vi "MAIN.vi"() -> ()   [LabVIEW 2021]
doc: "This is the main VI of the program. \n\nThis program required devices: the Power Meter (PM), the Stepper Motor (SM) and the Scannners."
uses:
  State.ctl
  State_2.ctl
  Data.ctl
  camera_data_cluster.ctl
  <vilib>/Utility/error.llb/DialogType.ctl
  <vilib>/DAQmx/write.llb/DAQmx Write (Analog 2D DBL NChan NSamp).vi
  <vilib>/DAQmx/read.llb/DAQmx Read (Digital Bool 1Line 1Point).vi
  <vilib>/DAQmx/create/channels.llb/DAQmx Create Channel (AO-Voltage-Basic).vi
  <vilib>/DAQmx/create/channels.llb/DAQmx Create Channel (DI-Digital Input).vi
  <vilib>/DAQmx/configure/timing.llb/DAQmx Timing (Sample Clock).vi
  <vilib>/DAQmx/miscellaneous.llb/DAQmx Fill In Error Info.vi
panel:
  out "Init filter position":sgl
  in  "Filter":bool
  out "FIX SM MotorRunState":i32(ring) items=["RunUnspecified", "RunStop", "RunForward", "RunReverse"]
  out "FIX SM CurrPosition":sgl
  out "FIX SM FaultStatus":bool
  out "IR SM MotorRunState":i32(ring) items=["RunUnspecified", "RunStop", "RunForward", "RunReverse"]
  out "IR SM CurrPosition":sgl
  out "IR SM FaultStatus":bool
  out "VIS SM MotorRunState":i32(ring) items=["RunUnspecified", "RunStop", "RunForward", "RunReverse"]
  out "VIS SM CurrPosition":sgl
  out "VIS SM FaultStatus":bool
  out "VIS GF MotorRunState":i32(ring) items=["RunUnspecified", "RunStop", "RunForward", "RunReverse"]
  out "VIS GF CurrPosition":sgl
  out "VIS GF FaultStatus":bool
  out "IR GF MotorRunState":i32(ring) items=["RunUnspecified", "RunStop", "RunForward", "RunReverse"]
  out "IR GF CurrPosition":sgl
  out "IR GF FaultStatus":bool
  out "Enum":T1=enum."Set power_1"
  in  "Threshold finding step [dB]":dbl=0.35 caption="Init power level [W]"
  in  "Investigated brightness range [dB]":sgl=10.0 caption="Init power level [W]"
  in  "Number of points M-2":i32=10 caption="Init power level [W]"
  in  "Number of trials k":i32=10 caption="Init power level [W]"
  out "Camera Image":picture
  out "Intensity graph output image":u8[][](graph) caption="Intensity Graph"
  out "error out 2":errorcluster
  out "loop down cond.":bool=TRUE
  out "loop up cond.":bool=TRUE
  out "Previous Position":i32=16
  in  "Save image?":bool
  out "#elements in queue":i32=2626
  out "Number of saved images":i32=2626
  in  "N_pts":u8=255
  in  "img_cols":u16=600
  in  "GB":u8=15
  in  "img_rows":u16=600
  in  "AT":u8=21
  in  "Auto gain":bool
  in  "Gain":i32(slide) scale=0.0..100.0
  in  "Frame rate":dbl(slide)=10.000850072256142 scale=9.830199684122917..40.10842644615945
  in  "Pixel clock":i32(slide)=24 scale=5.0..43.0
  in  "Exposure time":dbl(slide)=99.92475 scale=0.03841666666666667..99.96016666666667
  out "C brightness":bool[](array[boolean])
  out "Found?":bool[](array[boolean])=[TRUE, TRUE, TRUE, TRUE, TRUE, TRUE, TRUE, TRUE, TRUE, TRUE, TRUE, TRUE, TRUE, TRUE, TRUE, TRUE, TRUE]
  in  "Set Min Power [W]":dbl=8e-07 caption="Wavelength (0.0)" format="%#_6p"
  in  "Stop program":bool
  in  "Init power level [W]":dbl=0.0004 format="%#_6p"
  out "Measur. start time":timestamp=timestamp(3662016175.3575897 s since 1904-01-01)
  in  "Menu":enum32{"Test mode", "Measurement"}(tab)=enum."Measurement"
  in  "VIS SM GTP":bool
  in  "IR SM GTP":bool
  in  "FIX SM GTP":bool
  in  "VIS SM GTP":bool
  in  "IR SM GTP":bool
  in  "VIS GF GoToPos":sgl
  in  "IR GF GoToPos":sgl
  in  "FIX SM GoToPos":sgl
  in  "VIS SM GoToPos":sgl
  in  "IR SM GoToPos":sgl
  in  "Stimulus":bool
  in  "Illuminator OFF":bool
  in  "VIS br SM step [deg]":sgl
  in  "IR br SM step [deg]":sgl
  in  "FIX ref SM step [mm]":sgl
  in  "VIS ref SM step [mm]":sgl
  in  "IR ref SM step [mm]":sgl
  in  "VIS shutter":bool
  in  "IR shutter":bool
  in  "VIS brightness":bool
  in  "IR brightness":bool
  in  "FIX refraction SM":bool
  in  "VIS refraction SM":bool
  in  "IR refraction SM":bool
  in  "OK Button 2":bool
  in  "Set power [W]":dbl=6e-07 format="%#_6p"
  in  "FIX OFF":bool
  out "Test optotype":cluster{"sine wave":dbl[], "sine wave":dbl[]}(graph)={"sine wave"=[0.0, 0.002453383716370901, 0.0049008570164780305, 0.007336523722768088, 0.009754516100806413, 0.012149008995163194, 0.014514233862723118, 0.016844492669611, 0.019134171618254488, 0.021377754671514104, 0.02356983684129988, 0.025705137209661083, 0.02777851165098011, 0.029784965224621665, 0.03171966420818227, 0.03357794774235092, 0.035355339059327376, 0.03704755626774796, 0.038650522668136844, 0.04016037657403225, 0.04157348061512726, 0.04288643050001361, 0.04409606321741775, 0.045199464656172174, 0.046193976625564334, 0.047077203259151046, 0.047847016786610436, 0.04850156265972721, 0.04903926402016152, 0.04945882549823906, 0.04975923633360984, 0.04993977281025863, 0.049999999999999996, 0.04993977281025863, 0.04975923633360984, 0.04945882549823906, 0.04903926402016152, 0.04850156265972721, 0.047847016786610436, 0.047077203259151046, 0.04619397662556433, 0.045199464656172174, 0.04409606321741774, 0.04288643050001361, 0.04157348061512725, 0.04016037657403225, 0.03865052266813684, 0.03704755626774796, 0.03535533905932737, 0.03357794774235092, 0.03171966420818227, 0.029784965224621665, 0.02777851165098011, 0.025705137209661083, 0.02356983684129988, 0.0213777546715141, 0.019134171618254488, 0.016844492669610998, 0.014514233862723118, 0.012149008995163189, 0.009754516100806413, 0.007336523722768081, 0.00490085701647803, 0.002453383716370893, 0.0, -0.0024533837163709096, -0.00490085701647803, -0.007336523722768097, -0.009754516100806413, -0.012149008995163205, -0.014514233862723117, -0.016844492669611015, -0.019134171618254488, -0.021377754671514117, -0.02356983684129988, -0.0257051372096611, -0.02777851165098011, -0.029784965224621682, -0.03171966420818227, -0.033577947742350935, -0.03535533905932737, -0.03704755626774797, -0.03865052266813684, -0.040160376574032264, -0.04157348061512725, -0.042886430500013624, -0.04409606321741774, -0.04519946465617219, -0.04619397662556433, -0.04707720325915106, -0.047847016786610436, -0.04850156265972722, -0.04903926402016152, -0.04945882549823907, -0.04975923633360984, -0.049939772810258645, -0.049999999999999996, -0.049939772810258645, -0.04975923633360984, -0.04945882549823907, -0.04903926402016152, -0.04850156265972722, -0.047847016786610436, -0.04707720325915106, -0.04619397662556433, -0.04519946465617219, -0.04409606321741774, -0.042886430500013624, -0.04157348061512725, -0.040160376574032264, -0.03865052266813684, -0.03704755626774797, -0.03535533905932737, -0.033577947742350935, -0.03171966420818227, -0.02978496522462168, -0.02777851165098011, -0.025705137209661093, -0.02356983684129988, -0.021377754671514107, -0.019134171618254488, -0.016844492669611, -0.014514233862723118, -0.012149008995163189, -0.009754516100806413, -0.007336523722768078, -0.00490085701647803, -0.002453383716370887], "sine wave"=[0.05, 0.049939772810258624, 0.049759236333609846, 0.04945882549823905, 0.049039264020161524, 0.0485015626597272, 0.04784701678661044, 0.04707720325915104, 0.046193976625564334, 0.04519946465617217, 0.04409606321741775, 0.0428864305000136, 0.04157348061512726, 0.04016037657403224, 0.038650522668136844, 0.03704755626774795, 0.035355339059327376, 0.033577947742350914, 0.03171966420818227, 0.02978496522462166, 0.02777851165098011, 0.025705137209661083, 0.02356983684129988, 0.0213777546715141, 0.019134171618254488, 0.016844492669610998, 0.014514233862723117, 0.01214900899516319, 0.00975451610080641, 0.007336523722768084, 0.004900857016478025, 0.0024533837163708975, -6.071532165918825e-18, -0.0024533837163709035, -0.0049008570164780375, -0.00733652372276809, -0.009754516100806422, -0.012149008995163198, -0.014514233862723127, -0.016844492669611005, -0.019134171618254498, -0.021377754671514107, -0.023569836841299895, -0.025705137209661087, -0.027778511650980123, -0.029784965224621665, -0.031719664208182285, -0.033577947742350914, -0.03535533905932739, -0.037047556267747944, -0.03865052266813686, -0.040160376574032236, -0.04157348061512727, -0.042886430500013596, -0.04409606321741776, -0.04519946465617216, -0.04619397662556435, -0.04707720325915103, -0.04784701678661045, -0.048501562659727195, -0.04903926402016153, -0.049458825498239045, -0.04975923633360985, -0.04993977281025862, -0.05, -0.04993977281025862, -0.049759236333609846, -0.049458825498239045, -0.049039264020161524, -0.048501562659727195, -0.04784701678661044, -0.04707720325915103, -0.046193976625564334, -0.04519946465617216, -0.04409606321741775, -0.042886430500013596, -0.04157348061512726, -0.040160376574032236, -0.038650522668136844, -0.037047556267747944, -0.03535533905932737, -0.033577947742350914, -0.031719664208182265, -0.02978496522462166, -0.0277785116509801, -0.025705137209661083, -0.023569836841299867, -0.021377754671514104, -0.01913417161825447, -0.016844492669611, -0.0145142338627231, -0.012149008995163194, -0.009754516100806392, -0.007336523722768088, -0.004900857016478009, -0.002453383716370901, 2.168404344971009e-17, 0.0024533837163709, 0.004900857016478052, 0.007336523722768087, 0.009754516100806436, 0.012149008995163194, 0.01451423386272314, 0.016844492669611, 0.019134171618254512, 0.021377754671514104, 0.023569836841299905, 0.025705137209661083, 0.027778511650980133, 0.02978496522462166, 0.0317196642081823, 0.033577947742350914, 0.035355339059327404, 0.037047556267747944, 0.03865052266813687, 0.040160376574032236, 0.041573480615127285, 0.042886430500013596, 0.044096063217417776, 0.04519946465617216, 0.04619397662556436, 0.04707720325915103, 0.04784701678661046, 0.048501562659727195, 0.04903926402016154, 0.049458825498239045, 0.04975923633360986, 0.04993977281025862]}
  in  "Hide optotype":bool
  in  "X position":dbl
  in  "Select test optotype":u16(ring)=3 caption="Select optotype" items=["Circle", "Cross", "Square", "Flicker circle", "Beam", "Flicker beam"]
  in  "Y position":dbl
  in  "Size [V]":dbl=0.05 format="%#_13g"
  out "Threshold found?":bool
  out "Progress - found locations":u8(slide) max=5 step=1 scale=0.0..120.0
  in  "NO button":bool
  in  "YES button":bool
  out "Rate":dbl=12800.0
  in  "Min/Max Voltage":dbl=0.05 format="%#_13g"
  out "XY Graph":cluster{"sine wave":dbl[], "sine wave":dbl[]}(graph)={"sine wave"=[0.0, 0.002453383716370901, 0.0049008570164780305, 0.007336523722768088, 0.009754516100806413, 0.012149008995163194, 0.014514233862723118, 0.016844492669611, 0.019134171618254488, 0.021377754671514104, 0.02356983684129988, 0.025705137209661083, 0.02777851165098011, 0.029784965224621665, 0.03171966420818227, 0.03357794774235092, 0.035355339059327376, 0.03704755626774796, 0.038650522668136844, 0.04016037657403225, 0.04157348061512726, 0.04288643050001361, 0.04409606321741775, 0.045199464656172174, 0.046193976625564334, 0.047077203259151046, 0.047847016786610436, 0.04850156265972721, 0.04903926402016152, 0.04945882549823906, 0.04975923633360984, 0.04993977281025863, 0.049999999999999996, 0.04993977281025863, 0.04975923633360984, 0.04945882549823906, 0.04903926402016152, 0.04850156265972721, 0.047847016786610436, 0.047077203259151046, 0.04619397662556433, 0.045199464656172174, 0.04409606321741774, 0.04288643050001361, 0.04157348061512725, 0.04016037657403225, 0.03865052266813684, 0.03704755626774796, 0.03535533905932737, 0.03357794774235092, 0.03171966420818227, 0.029784965224621665, 0.02777851165098011, 0.025705137209661083, 0.02356983684129988, 0.0213777546715141, 0.019134171618254488, 0.016844492669610998, 0.014514233862723118, 0.012149008995163189, 0.009754516100806413, 0.007336523722768081, 0.00490085701647803, 0.002453383716370893, 0.0, -0.0024533837163709096, -0.00490085701647803, -0.007336523722768097, -0.009754516100806413, -0.012149008995163205, -0.014514233862723117, -0.016844492669611015, -0.019134171618254488, -0.021377754671514117, -0.02356983684129988, -0.0257051372096611, -0.02777851165098011, -0.029784965224621682, -0.03171966420818227, -0.033577947742350935, -0.03535533905932737, -0.03704755626774797, -0.03865052266813684, -0.040160376574032264, -0.04157348061512725, -0.042886430500013624, -0.04409606321741774, -0.04519946465617219, -0.04619397662556433, -0.04707720325915106, -0.047847016786610436, -0.04850156265972722, -0.04903926402016152, -0.04945882549823907, -0.04975923633360984, -0.049939772810258645, -0.049999999999999996, -0.049939772810258645, -0.04975923633360984, -0.04945882549823907, -0.04903926402016152, -0.04850156265972722, -0.047847016786610436, -0.04707720325915106, -0.04619397662556433, -0.04519946465617219, -0.04409606321741774, -0.042886430500013624, -0.04157348061512725, -0.040160376574032264, -0.03865052266813684, -0.03704755626774797, -0.03535533905932737, -0.033577947742350935, -0.03171966420818227, -0.02978496522462168, -0.02777851165098011, -0.025705137209661093, -0.02356983684129988, -0.021377754671514107, -0.019134171618254488, -0.016844492669611, -0.014514233862723118, -0.012149008995163189, -0.009754516100806413, -0.007336523722768078, -0.00490085701647803, -0.002453383716370887], "sine wave"=[0.05, 0.049939772810258624, 0.049759236333609846, 0.04945882549823905, 0.049039264020161524, 0.0485015626597272, 0.04784701678661044, 0.04707720325915104, 0.046193976625564334, 0.04519946465617217, 0.04409606321741775, 0.0428864305000136, 0.04157348061512726, 0.04016037657403224, 0.038650522668136844, 0.03704755626774795, 0.035355339059327376, 0.033577947742350914, 0.03171966420818227, 0.02978496522462166, 0.02777851165098011, 0.025705137209661083, 0.02356983684129988, 0.0213777546715141, 0.019134171618254488, 0.016844492669610998, 0.014514233862723117, 0.01214900899516319, 0.00975451610080641, 0.007336523722768084, 0.004900857016478025, 0.0024533837163708975, -6.071532165918825e-18, -0.0024533837163709035, -0.0049008570164780375, -0.00733652372276809, -0.009754516100806422, -0.012149008995163198, -0.014514233862723127, -0.016844492669611005, -0.019134171618254498, -0.021377754671514107, -0.023569836841299895, -0.025705137209661087, -0.027778511650980123, -0.029784965224621665, -0.031719664208182285, -0.033577947742350914, -0.03535533905932739, -0.037047556267747944, -0.03865052266813686, -0.040160376574032236, -0.04157348061512727, -0.042886430500013596, -0.04409606321741776, -0.04519946465617216, -0.04619397662556435, -0.04707720325915103, -0.04784701678661045, -0.048501562659727195, -0.04903926402016153, -0.049458825498239045, -0.04975923633360985, -0.04993977281025862, -0.05, -0.04993977281025862, -0.049759236333609846, -0.049458825498239045, -0.049039264020161524, -0.048501562659727195, -0.04784701678661044, -0.04707720325915103, -0.046193976625564334, -0.04519946465617216, -0.04409606321741775, -0.042886430500013596, -0.04157348061512726, -0.040160376574032236, -0.038650522668136844, -0.037047556267747944, -0.03535533905932737, -0.033577947742350914, -0.031719664208182265, -0.02978496522462166, -0.0277785116509801, -0.025705137209661083, -0.023569836841299867, -0.021377754671514104, -0.01913417161825447, -0.016844492669611, -0.0145142338627231, -0.012149008995163194, -0.009754516100806392, -0.007336523722768088, -0.004900857016478009, -0.002453383716370901, 2.168404344971009e-17, 0.0024533837163709, 0.004900857016478052, 0.007336523722768087, 0.009754516100806436, 0.012149008995163194, 0.01451423386272314, 0.016844492669611, 0.019134171618254512, 0.021377754671514104, 0.023569836841299905, 0.025705137209661083, 0.027778511650980133, 0.02978496522462166, 0.0317196642081823, 0.033577947742350914, 0.035355339059327404, 0.037047556267747944, 0.03865052266813687, 0.040160376574032236, 0.041573480615127285, 0.042886430500013596, 0.044096063217417776, 0.04519946465617216, 0.04619397662556436, 0.04707720325915103, 0.04784701678661046, 0.048501562659727195, 0.04903926402016154, 0.049458825498239045, 0.04975923633360986, 0.04993977281025862]}
  in  "Select optotype":u16(ring)=3 items=["Circle", "Cross", "Square", "Flicker circle", "Beam", "Flicker beam"]
  in  "shiftX":dbl
  in  "shiftY":dbl
  in  "Start measurement":bool
  in  "Pause":bool
  out "Answers":i32[][](array[numeric])
  out "Previous brightess":i32
  out "Filter positions [deg]":sgl[](array[numeric])
  out "Progress - found locations 2":u8 max=5 step=1
  in  "Set Max Power [W]":dbl=0.0004 caption="Wavelength (0.0)" format="%#_6p"
  out "Patient button":bool
  out "Any USB device connected?":bool=TRUE
  in  "Set Wavelength [nm]":dbl=1040.0 caption="Wavelength (0.0)"
  out "Current position [steps]":i32
  in  "File Path":path=path "D:/meas_data"
  out "Power Value":dbl=4.76676519e-07 caption="Optical Power [W]" format="%#_4p"
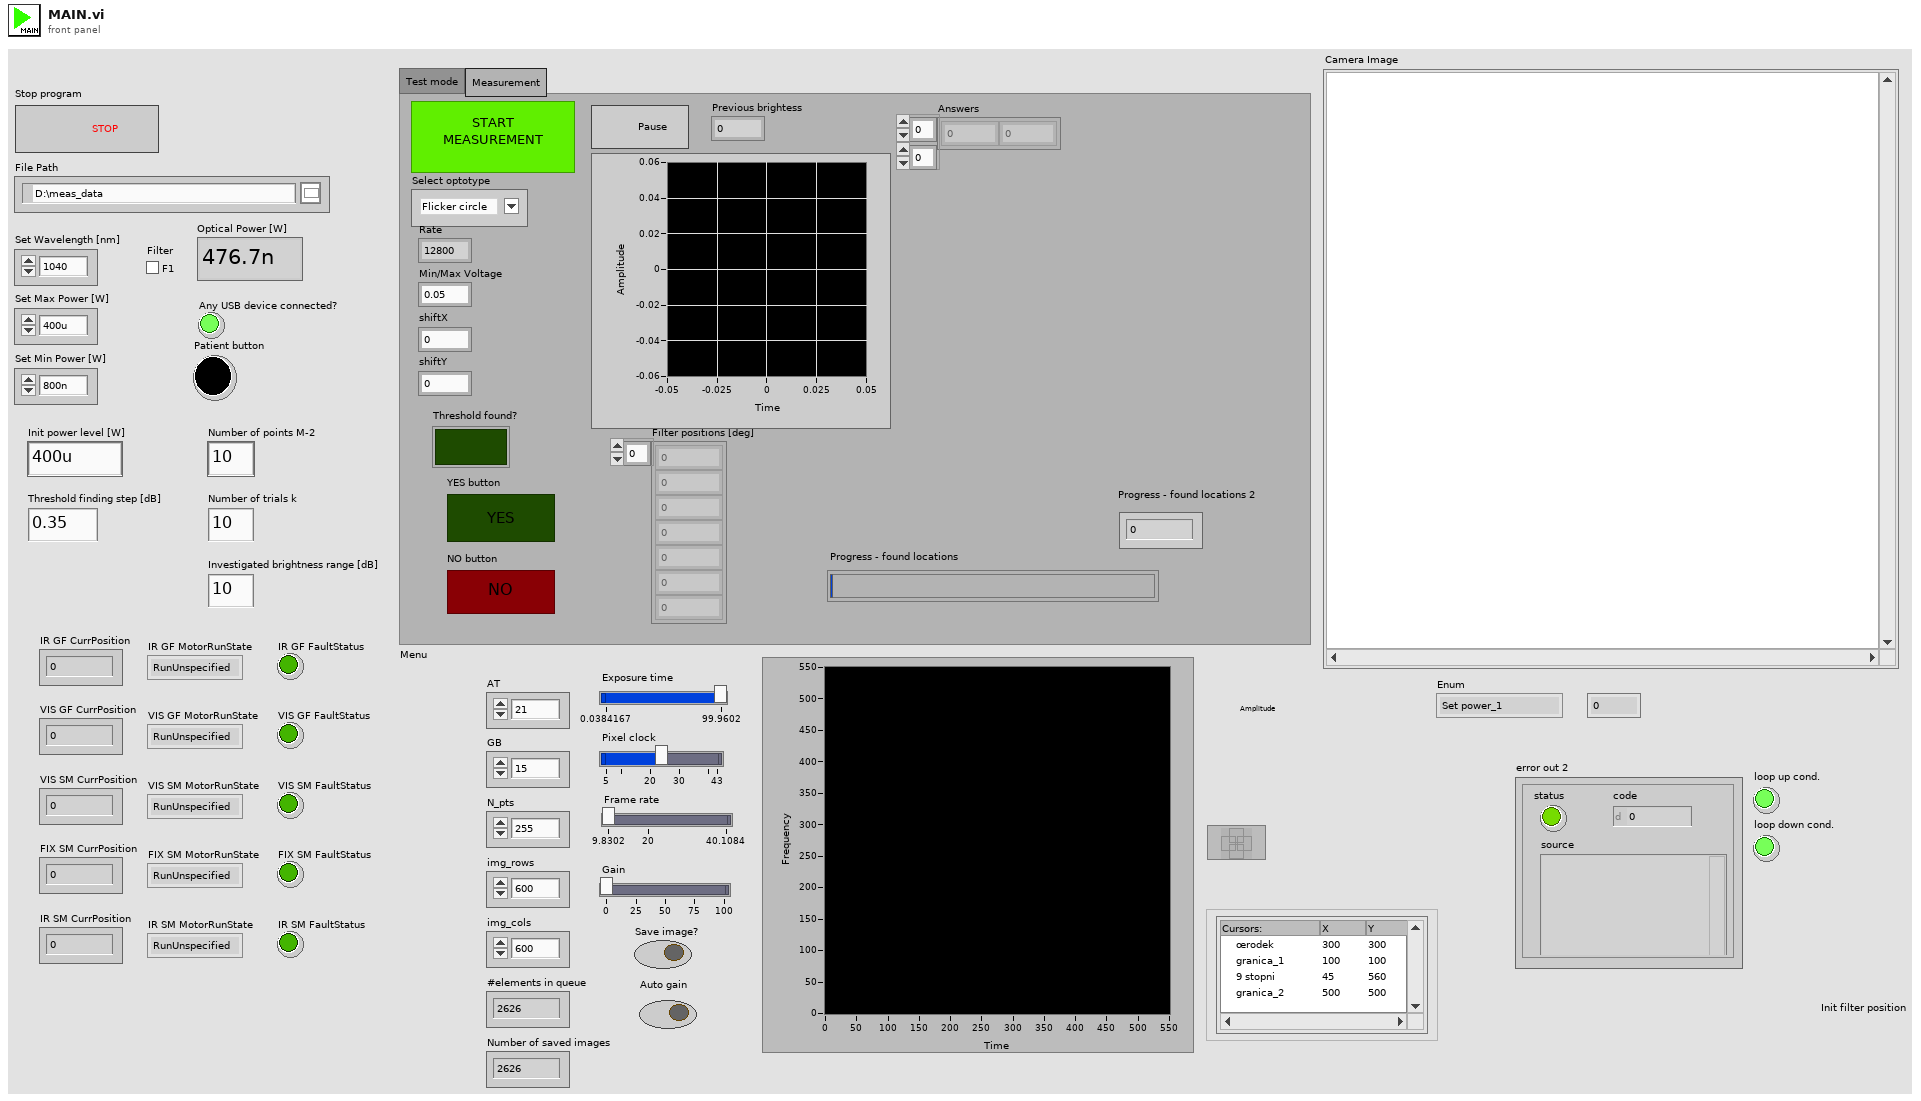
[diagram p1: front panel]
types:
  T1 = typedef "State.ctl" = enum16{"Initialize", "Idle_2", "Random brightness", "Hide optotype_2", "Hide optotype_1", "Set power_1", "Set_power_2", "Show optotype", "Wait for event", "Yes_1", "Yes_2", "No_2", "No_1", "Idle_1", "Exit"}
  T2 = typedef "Data.ctl" = cluster{cluster{"Power [W]":dbl, "Position":string, "Answer":string, "Seconds form start [s]":dbl, "Time stamp":timestamp}}[]
  T3 = typedef "State_2.ctl" = enum16{"Wait for event", "Set power", "Update optotype"}
  T4 = typedef "camera_data_cluster.ctl" = cluster{"Time stamp":timestamp, "Image":u8[][], "Z Scale.Range:Maximum":dbl, "Z Scale.Range:Minimum":dbl, "Color Table":u32[]}
  T5 = cluster{"s32Width":i32, "s32PosX":i32, "s32PosY":i32, "s32PosY":i32}
  T6 = cluster{"Power Value":dbl, string, string, dbl, "seconds since 1Jan1904":timestamp}
  T7 = cluster{cluster{"Power Value":dbl, string, string, dbl, "seconds since 1Jan1904":timestamp}}[]
  T8 = cluster{"Pixel clock":refnum<vi>, "Frame rate":refnum<vi>, "Exposure time":refnum<vi>, "Gain":refnum<vi>, "Auto gain":bool}
  T9 = cluster{"img_rows":u16, "img_cols":u16, "AT":u8, "GB":u8, "N_pts":u8}
  T10 = typedef "DialogType.ctl" = u16
  T11 = cluster{"Set Wavelength [nm]":dbl, "Min/Max Voltage":dbl, "shiftX":dbl, "shiftY":dbl, "Filter positions [deg]":sgl[], "Answers":i32[][]}
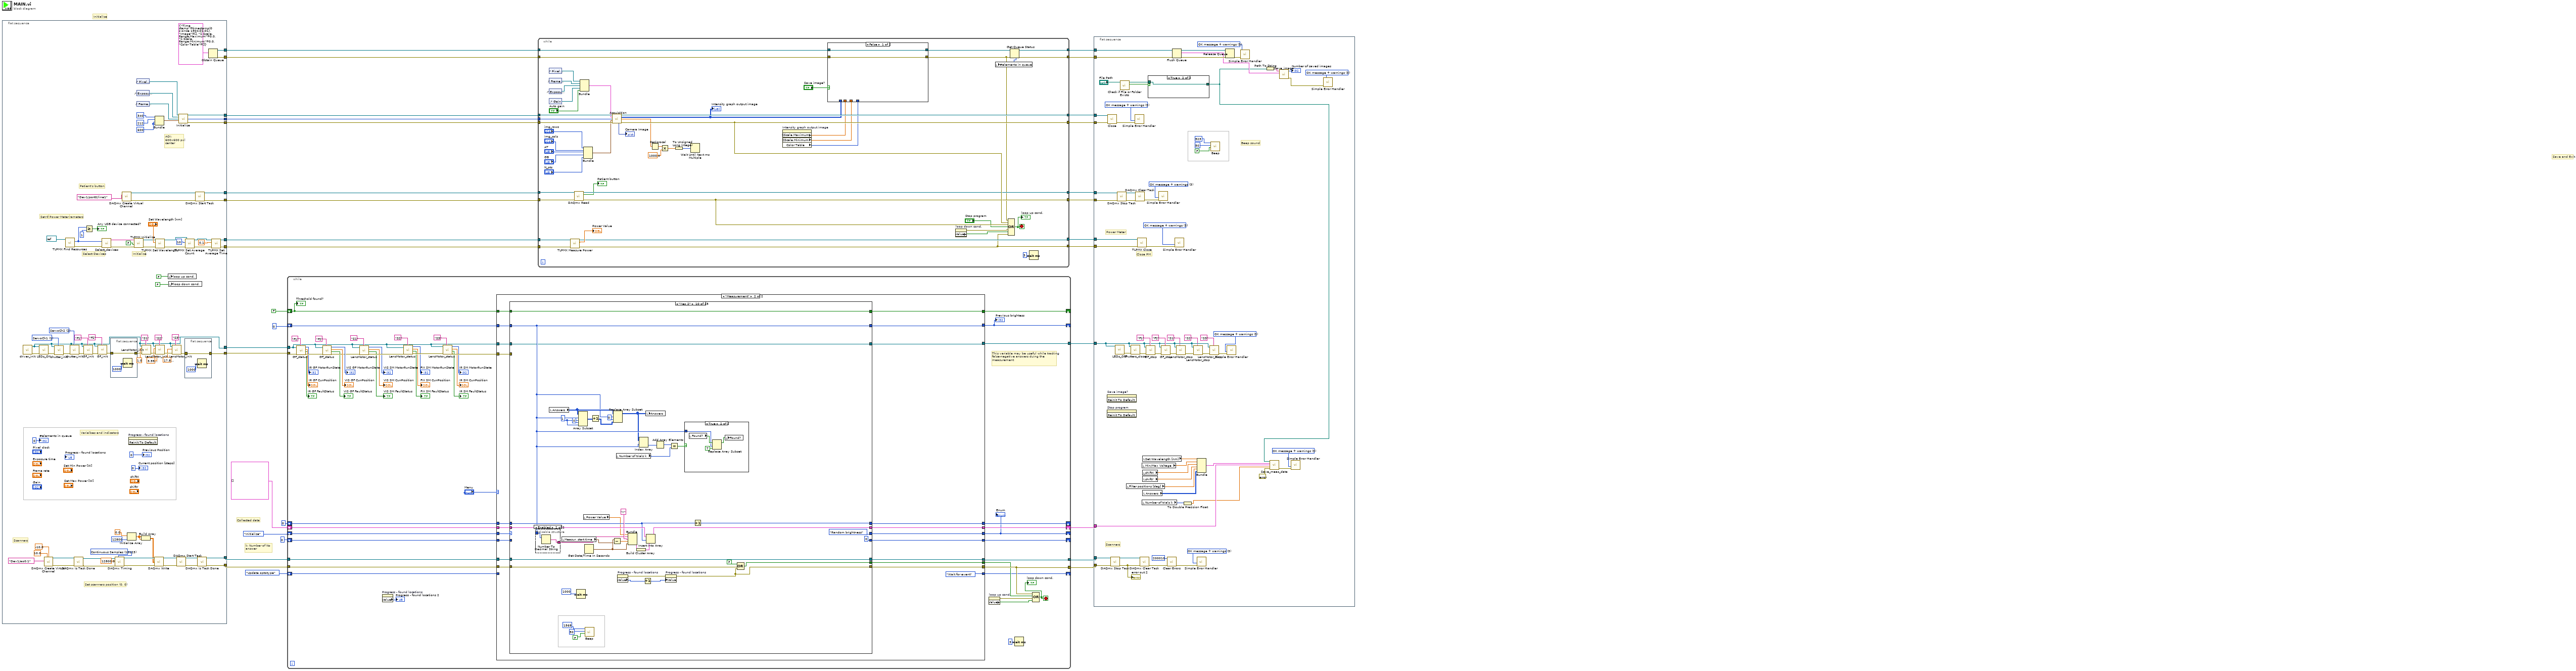
[diagram p0: block diagram]
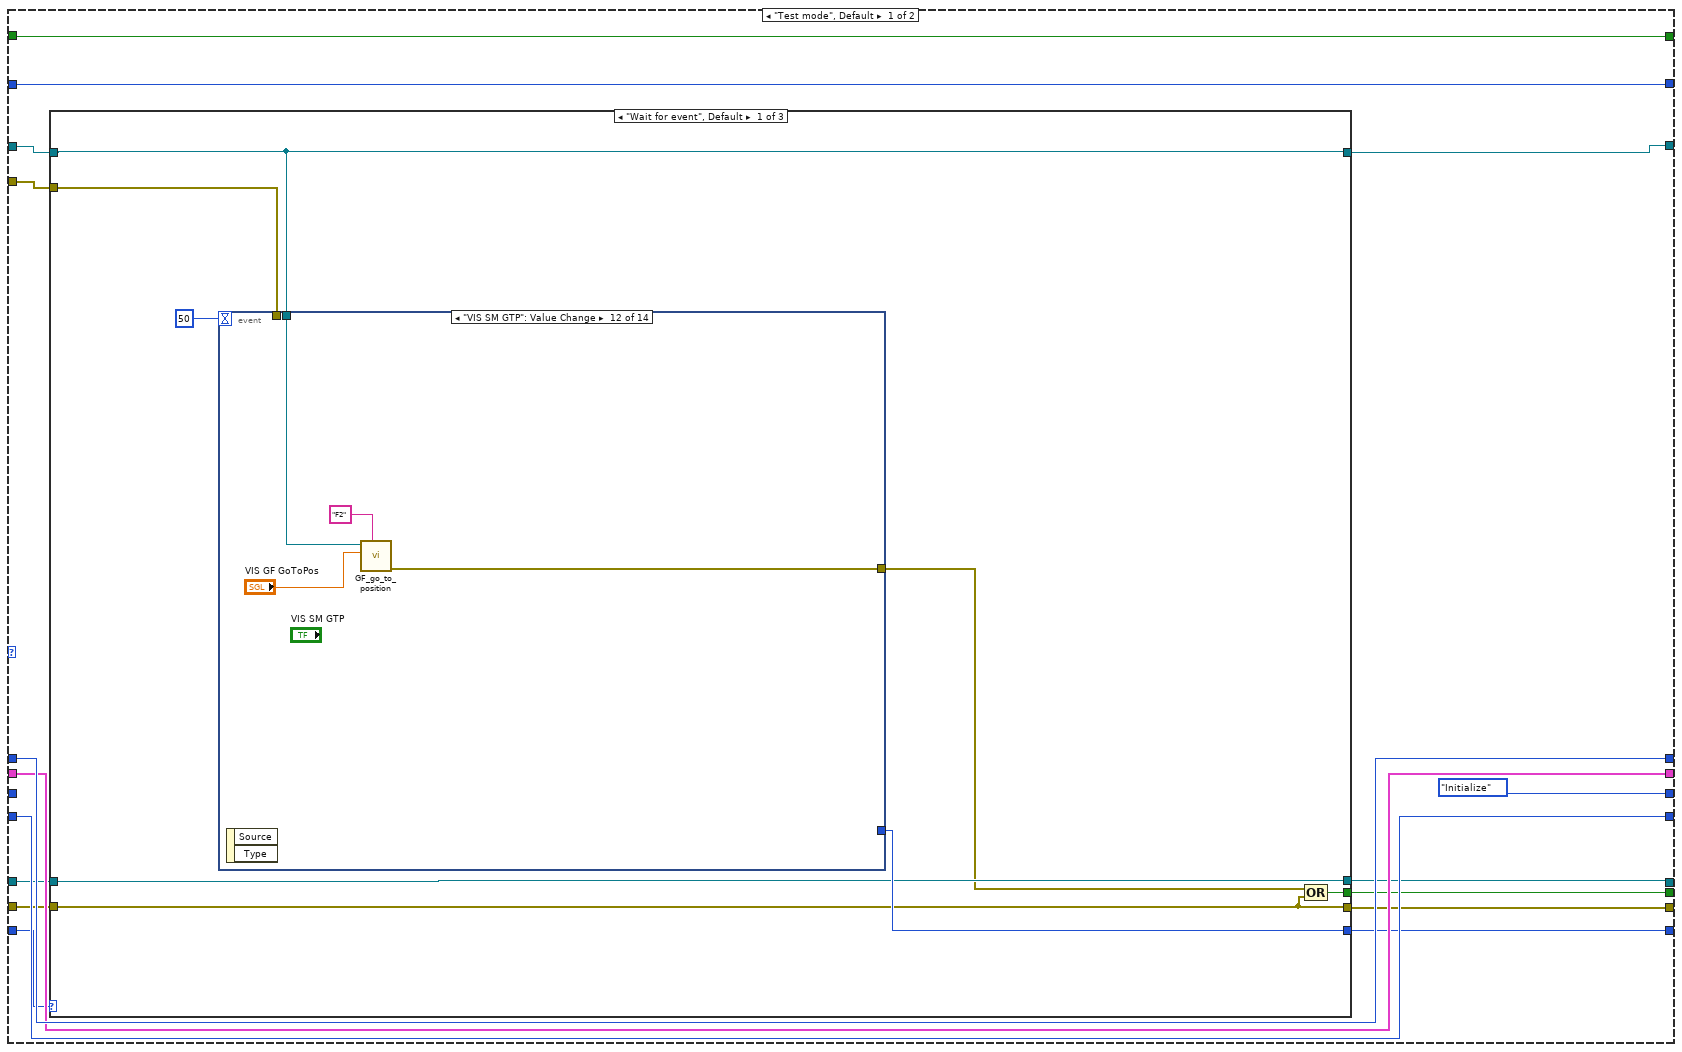
[diagram p2: hidden frame]
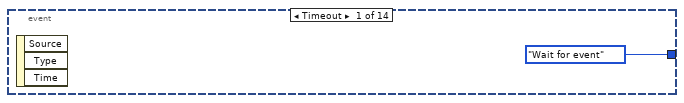
[diagram p3: hidden frame]
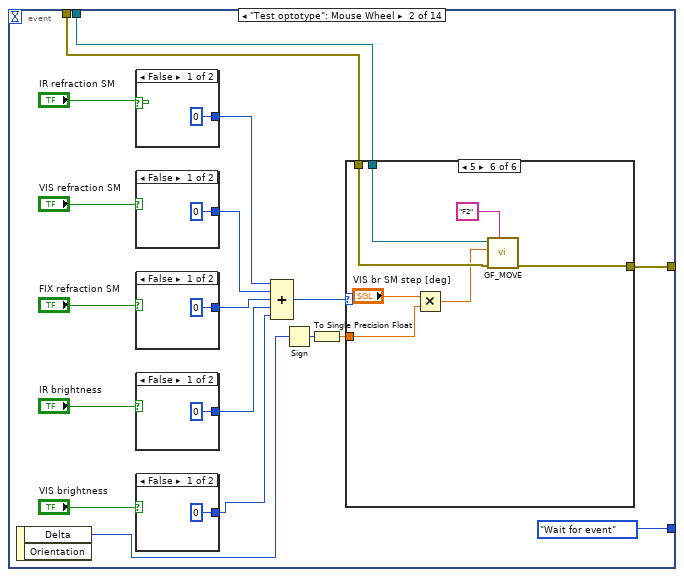
[diagram p4: hidden frame]
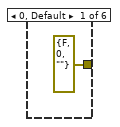
[diagram p5: hidden frame]
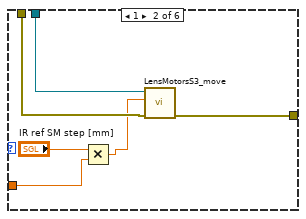
[diagram p6: hidden frame]
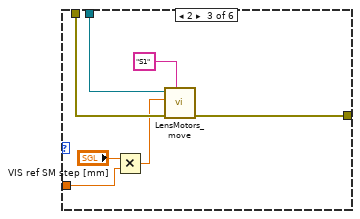
[diagram p7: hidden frame]
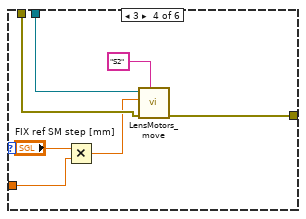
[diagram p8: hidden frame]
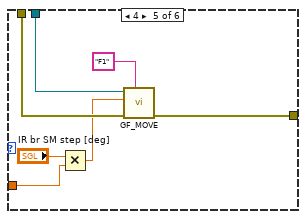
[diagram p9: hidden frame]
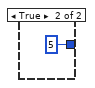
[diagram p10: hidden frame]
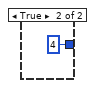
[diagram p11: hidden frame]
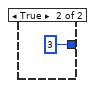
[diagram p12: hidden frame]
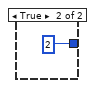
[diagram p13: hidden frame]
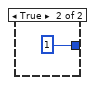
[diagram p14: hidden frame]
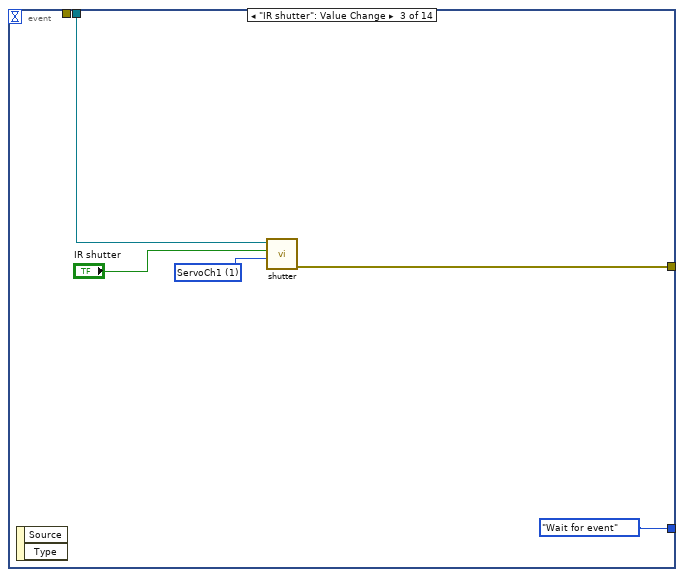
[diagram p15: hidden frame]
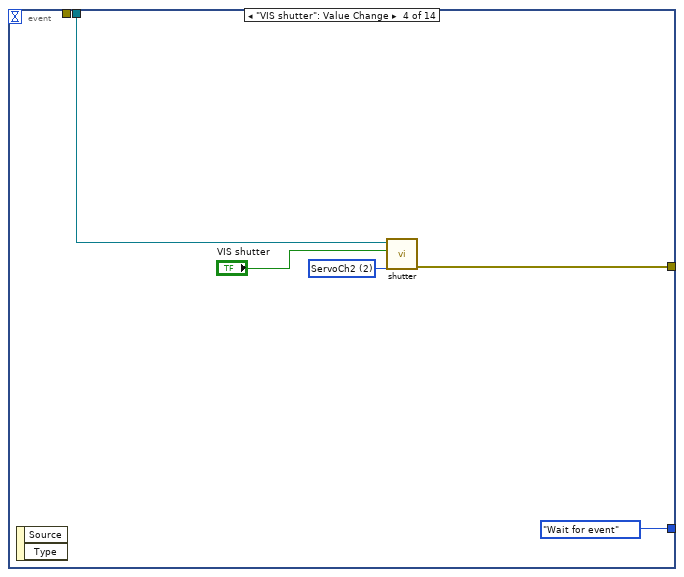
[diagram p16: hidden frame]
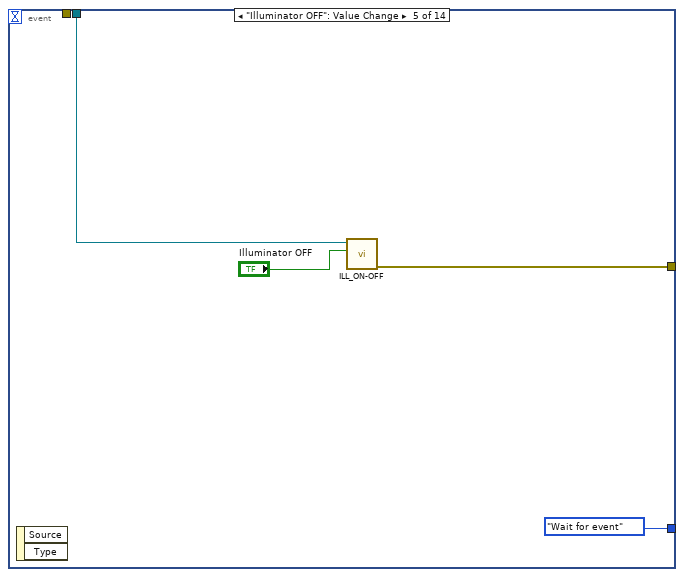
[diagram p17: hidden frame]
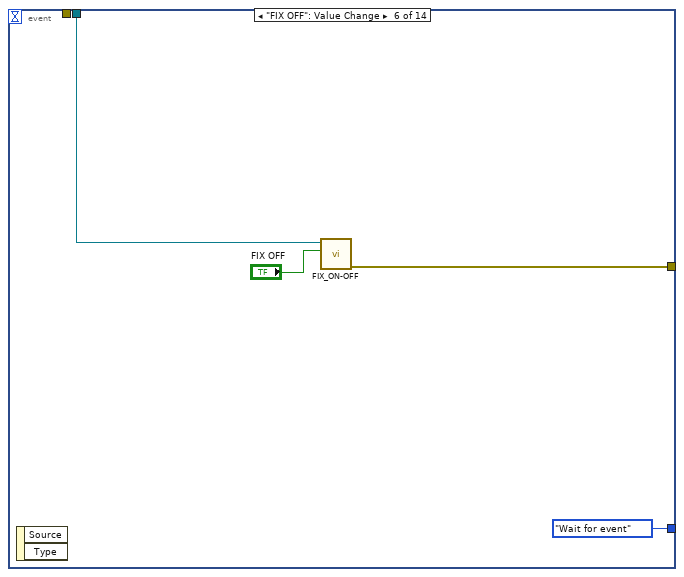
[diagram p18: hidden frame]
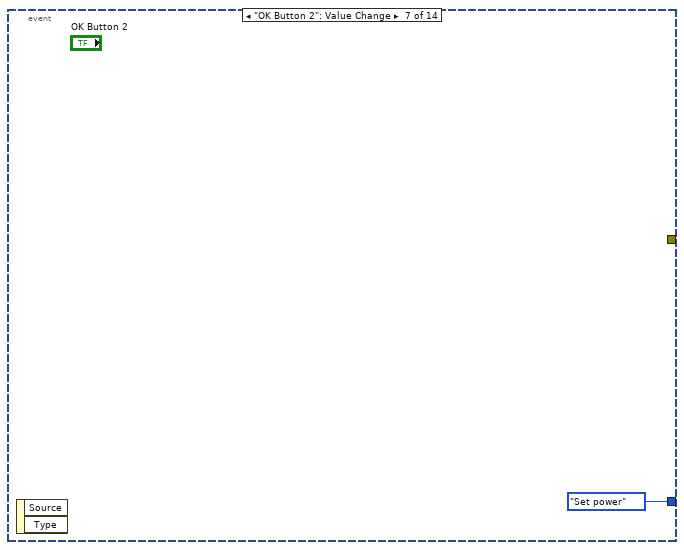
[diagram p19: hidden frame]
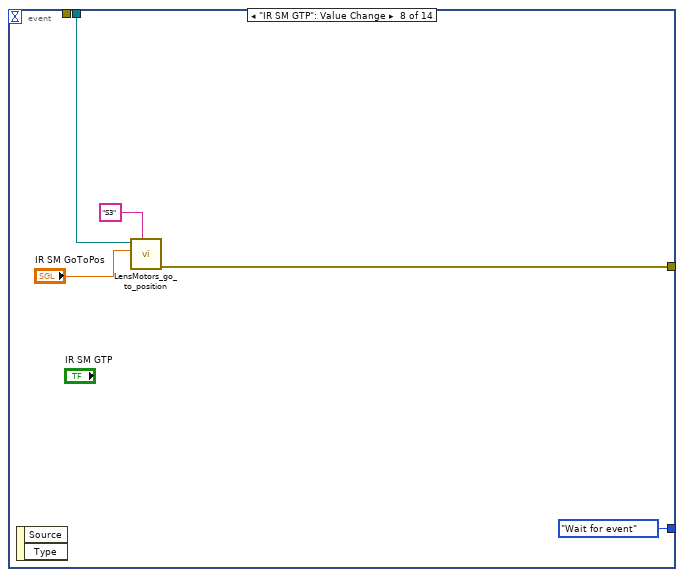
[diagram p20: hidden frame]
diagram:
  # "k: Number of No\nanswer"
  # "Collected data"
  # "Save and Exit"
  # "Initialize"
  n1 = flat-sequence {
    tunnel: [w117] -> w28
    tunnel: [w116] -> w27
    tunnel: [w115] -> w26
    tunnel: [w114] -> w23
    tunnel: [w113] -> w22
    tunnel: [w112] -> w21
    tunnel: [w111] -> w15
    tunnel: [w86] -> w14
    tunnel: [w85] -> w13
    tunnel: [w39] -> w5
    tunnel: [w40] -> w4
    tunnel: [w51] -> w3
    tunnel: [w50] -> w2
    frame #0 {
      w67 = 2 items=["ServoUnspecified", "ServoCh1", "ServoCh2", "ServoBoth"] ("servo")
      w68 = 1 items=["ServoUnspecified", "ServoCh1", "ServoCh2", "ServoBoth"] ("servo")
      w72 = 600 ("s32PosY")
      w94 = 10123 items=["Finite Samples"=10178, "Continuous Samples"=10123, "Hardware Timed Single Point"=12522] ("sample mode")
      # "Set the SM start parameters"
      # "AOI:\n600x600 pxl\ncenter"
      # "Set scanners position (0, 0)"
      # "Patient's button"
      # "Scanners"
      # "Power Meter"
      # "Initialize"
      # "Select Devices"
      # "Varialbes and indicators"
      n2 = call "driver_init.vi"() -> ("error out"=w71:errorcluster, "new reference"=w50:refnum<k24>)  [unwired: 10 in]
      n3 = call "LEDs_ON.vi"("error in (no error)"=w71, "channel"=w50) -> ("error out"=w70:errorcluster)  [unwired: 9 in]
      n4 = call-poly <vilib>:"DAQmx Create Virtual Channel.vi"("maximum value"=10.0, "minimum value"=-10.0, "physical channels"=tag "Dev1/ao0:1") -> ("task out"=w96:refnum<k21>, "error out"=w95:errorcluster)  [unwired: 11 in]
      n5 = call "shutter_init.vi"("servo"=w68, "error in (no error)"=w70, "channel"=w50) -> ("error out"=w69:errorcluster)  [unwired: 8 in]
      n6 = call "TLPMX Find Resources.vi"("instrument handle"=refnum<visa-resource-name> refnum) -> ("error out"=w49:errorcluster, "Resource Count"=w48:u32)  [unwired: 8 in, 1 out]
      n7 = call "shutter_init.vi"("servo"=w67, "error in (no error)"=w69, "channel"=w50) -> ("error out"=w66:errorcluster)  [unwired: 8 in]
      n8 = call <vilib>:"DAQmx Is Task Done.vi"("task/channels in"=w96, "error in"=w95) -> ("task out"=w93:refnum<k21>, "error out"=w92:errorcluster)  [unwired: 11 in, 1 out]
      n9 = call "GF_init.vi"("modIdTag"="F1", "error in (no error)"=w66, "channel"=w50) -> ("error out"=w65:errorcluster)  [unwired: 8 in]
      n10 = Greater Or Equal?(x=w48, y=u32 1) -> (x >= y?=→"Any USB device connected?":bool)
      n11 = call "GF_init.vi"("modIdTag"="F2", "error in (no error)"=w65, "channel"=w50) -> ("error out"=w62:errorcluster)  [unwired: 8 in]
      n12 = call "Select_devices.vi"("error in (no error)"=w49, "Number of devices"=w48) -> ("error out"=w44:errorcluster, "PM ResourceName Out"=w46:string)  [unwired: 8 in]
      n13 = flat-sequence {
        tunnel: w62 -> [w120]
        tunnel: [w120] -> w61
        frame #0 {
          n14 = Wait (ms)(milliseconds to wait=u32 1000) -> ()  [unwired: 1 out]
        }
      }
      n15 = call-poly <vilib>:"DAQmx Timing.vi"("task/channels in"=w93, "sample mode"=w94, "rate"=12800.0, "error in"=w92) -> ("task out"=w104:refnum<k21>, "error out"=w102:errorcluster)  [unwired: 10 in]
      n16 = call-poly <vilib>:"DAQmx Create Virtual Channel.vi"("lines"=tag "Dev1/port0/line1" ("Line(s)")) -> ("task out"=w83:refnum<k21>, "error out"=w82:errorcluster)  [unwired: 13 in]
      n17 = Initialize Array(0.0 ("element"), 12800 ("dimension size")) -> (w89:dbl[])
      n18 = invoke on="Progress - found locations" class="Slide (strict)" method="Reinit To Default"() -> ()  [unwired: 3 in, 3 out]
      n19 = call "TLPMX Initialize.vi"("error in (no error)"=w44, "Reset Device (Yes)"=FALSE ("ID Query (Do Query)"), "resource name"=w46) -> ("error out"=w43:errorcluster, "instrument handle out"=w41:refnum<visa-resource-name>)  [unwired: 7 in]
      n20 = control-ref of="Pixel clock"() -> (w78:refnum<vi>)
      n21 = control-ref of="Exposure time"() -> (w77:refnum<vi>)
      n22 = control-ref of="Frame rate"() -> (w76:refnum<vi>)
      n23 = Build Array(w89, w89) -> (w101:dbl[][])
      n24 = call "LensMotor_init.vi"("modIdTag"="S1", "error in (no error)"=w61, "position"=sgl 1.0, "channel"=w50) -> ("error out"=w60:errorcluster)  [unwired: 7 in]
      n25 = call-poly <vilib>:"DAQmx Write.vi"("task/channels in"=w104, "data"=w101, "error in"=w102) -> ("task out"=w100:refnum<k21>, "error out"=w99:errorcluster)  [unwired: 10 in, 1 out]
      n26 = Bundle("s32Width"=340, "s32PosX"=212, "s32PosY"=w72, "s32PosY"=w72) -> (w75:T5)  [unwired: 1 in]
      n27 = call "TLPMX Set Wavelength.vi"("error in (no error)"=w43, "Wavelength (0.0)"="Set Wavelength [nm]", "instrument handle"=w41) -> ("error out"=w38:errorcluster, "instrument handle out"=w37:refnum<visa-resource-name>)  [unwired: 7 in]
      n28 = call "LensMotor_init.vi"("modIdTag"="S2", "error in (no error)"=w60, "position"=sgl 3.99, "channel"=w50) -> ("error out"=w59:errorcluster)  [unwired: 7 in]
      n29 = local write "loop up cond."(FALSE ("result loop 1")) -> ()
      n30 = local write "loop down cond."(FALSE ("result loop 2")) -> ()
      n31 = call "LensMotor_init.vi"("modIdTag"="S3", "error in (no error)"=w59, "position"=sgl 17.9, "channel"=w50) -> ("error out"=w52:errorcluster)  [unwired: 7 in]
      n32 = call <vilib>:"DAQmx Start Task.vi"("task/channels in"=w100, "error in"=w99) -> ("task out"=w91:refnum<k21>, "error out"=w90:errorcluster)  [unwired: 12 in]
      n33 = call "Initialize.vi"("Get PxlClk Slide"=w78, "Get Expos Slide"=w77, "Get FPS Slide"=w76, "ROI Data Cluster"=w75) -> ("uc480.Camera"=w111:refnum<k24>, "Bits/Pixel 2"=w114:i32, "Error Out"=w115:errorcluster)  [unwired: 8 in, 1 out]
      n34 = flat-sequence {
        tunnel: w52 -> [w118]
        tunnel: [w118] -> w51
        frame #0 {
          n35 = Wait (ms)(milliseconds to wait=u32 1000) -> ()  [unwired: 1 out]
        }
      }
      n36 = call "TLPMX Set Average Count.vi"("error in (no error)"=w38, "Average Count (1)"=i16 10, "instrument handle"=w37) -> ("error out"=w35:errorcluster, "instrument handle out"=w34:refnum<visa-resource-name>)  [unwired: 7 in]
      n37 = call <vilib>:"DAQmx Start Task.vi"("task/channels in"=w83, "error in"=w82) -> ("task out"=w86:refnum<k21>, "error out"=w85:errorcluster)  [unwired: 12 in]
      n38 = call <vilib>:"DAQmx Is Task Done.vi"("task/channels in"=w91, "error in"=w90) -> ("task out"=w117:refnum<k21>, "error out"=w116:errorcluster)  [unwired: 11 in, 1 out]
      n39 = Obtain Queue(element data type=T4 {"Time stamp"=timestamp(0 s since 1904-01-01), "Image"=[], "Z Scale.Range:Maximum"=0.0, "Z Scale.Range:Minimum"=0.0, "Color Table"=[]}) -> (queue out=w113:refnum<queue>, error out=w112:errorcluster)  [unwired: 4 in, 1 out]
      n40 = call "TLPMX Set Average Time.vi"("error in (no error)"=w35, "Average Time (0.0)"=0.1, "instrument handle"=w34) -> ("error out"=w40:errorcluster, "instrument handle out"=w39:refnum<visa-resource-name>)  [unwired: 7 in]
      "Current position [steps]" <- 0
      "#elements in queue" <- 0 ("#elements in queue")
      "Previous Position" <- 0
    }
  }
  n41 = while {
    shift-right: [w161] -> _
    shift-left: State_2."Update optotype" ("Enum") -> [w167]
    shift-right: [w162] -> _
    shift-left: 0 -> [w169]
    shift-right: [w155] -> _
    shift-left: State."Initialize" -> [w156]
    shift-right: [w163] -> _
    shift-left: 0 -> [w168]
    tunnel: w27 -> [w171]
    tunnel: [w174] -> w30
    tunnel: w28 -> [w172]
    tunnel: [w173] -> w29
    shift-right: [w159] -> w9
    shift-left: T2 [] ("Data") -> [w170]
    shift-right: [w157] -> _
    shift-left: 0 -> [w158]
    shift-right: [w153] -> _
    shift-left: FALSE -> [w154]
    tunnel: w3 -> [w152]
    tunnel: w2 -> [w126]
    tunnel: [w125] -> w1
    stop <- w160 stop-if-true
    # "This variable may be useful while tracking false-negative answers duing the measurement"
    n42 = call "GF_status.vi"("modIdTag"="F1", "error in (no error)"=w152, "channel"=w126) -> ("error out"=w150:errorcluster, "MotorFaultStatus"=→"IR GF FaultStatus":bool, "CurrPosition"=→"IR GF CurrPosition":sgl, "MotorRunState"=→"IR GF MotorRunState":i32)  [unwired: 5 in]
    n43 = call "GF_status.vi"("modIdTag"="F2", "error in (no error)"=w150, "channel"=w126) -> ("error out"=w142:errorcluster, "MotorFaultStatus"=→"VIS GF FaultStatus":bool, "CurrPosition"=→"VIS GF CurrPosition":sgl, "MotorRunState"=→"VIS GF MotorRunState":i32)  [unwired: 5 in]
    n44 = call "LensMotor_status.vi"("modIdTag"="S1", "error in (no error)"=w142, "channel"=w126) -> ("error out"=w151:errorcluster, "MotorFaultStatus"=→"VIS SM FaultStatus":bool, "CurrPosition"=→"VIS SM CurrPosition":sgl, "MotorRunState"=→"VIS SM MotorRunState":i32)  [unwired: 5 in]
    n45 = property on="Progress - found locations" class="Slide (strict)"() -> ("Value"=→"Progress - found locations 2":u8)  [unwired: 2 in, 2 out]
    n46 = call "LensMotor_status.vi"("modIdTag"="S2", "error in (no error)"=w151, "channel"=w126) -> ("error out"=w139:errorcluster, "MotorFaultStatus"=→"FIX SM FaultStatus":bool, "CurrPosition"=→"FIX SM CurrPosition":sgl, "MotorRunState"=→"FIX SM MotorRunState":i32)  [unwired: 5 in]
    n47 = call "LensMotor_status.vi"("modIdTag"="S3", "error in (no error)"=w139, "channel"=w126) -> ("error out"=w130:errorcluster, "MotorFaultStatus"=→"IR SM FaultStatus":bool, "CurrPosition"=→"IR SM CurrPosition":sgl, "MotorRunState"=→"IR SM MotorRunState":i32)  [unwired: 5 in]
    n48 = case shown="\"Measurement\"" "Menu" {
      tunnel: w172 -> [w185 w428]
      tunnel: w171 -> [w183 w427]
      tunnel: [w181 w426] -> w165
      tunnel: w169 -> [w189 w425]
      tunnel: [w189 w424] -> w162
      tunnel: [w190 w423] -> w163
      tunnel: w170 -> [w188 w422]
      tunnel: w168 -> [w190 w421]
      tunnel: [w188 w420] -> w159
      tunnel: [w184 w419] -> w173
      tunnel: [w182 w418] -> w174
      tunnel: w167 -> [w187 _]
      tunnel: [w186 State_2."Wait for event" ("Enum")] -> w161
      tunnel: [w180 w416] -> w157
      tunnel: w158 -> [w180 w415]
      tunnel: w156 -> [_ w414]
      tunnel: [State."Initialize" w413] -> w155
      tunnel: w154 -> [w178 w412]
      tunnel: [w178 w411] -> w153
      tunnel: w130 -> [w175 w410]
      tunnel: w126 -> [w177 w409]
      tunnel: [w176 w408] -> w125
      frame "Test mode", Default {
        n49 = case shown="\"Wait for event\", Default" w187 {
          tunnel: [w198 w313 State_2."Wait for event" ("Enum")] -> w186
          tunnel: w185 -> [w195 w326 w352]
          tunnel: [w195 w326 w350] -> w184
          tunnel: w183 -> [w194 w324 w351]
          tunnel: [w194 w324 w348] -> w182
          tunnel: [w196 w325 w347] -> w181
          tunnel: w177 -> [w192 w306 w345]
          tunnel: [w192 w306 w345] -> w176
          tunnel: w175 -> [w191 _ _]
          frame "Wait for event", Default {
            n50 = event shown="[11] \"VIS SM GTP\": Value Change" {
              selector: _ -> [_ _ _ _ _ _ _ _ _ _ _ _ _ _]
              dyn-events: _ -> [_ _ _ _ _ _ _ _ _ _ _ _ _ _]
              timeout: 50 -> [_ _ _ _ _ _ _ _ _ _ _ _ _ _]
              tunnel: [State_2."Wait for event" ("Enum") State_2."Wait for event" ("Enum") State_2."Wait for event" ("Enum") State_2."Wait for event" ("Enum") State_2."Wait for event" ("Enum") State_2."Wait for event" ("Enum") State_2."Set power" ("Enum") State_2."Wait for event" ("Enum") _ _ _ _ State_2."Update optotype" ("Enum") State_2."Update optotype" ("Enum")] -> w198
              tunnel: w192 -> [_ w205 w265 w272 w274 w278 _ w286 w289 w293 w297 w301 _ _]
              tunnel: [_ w204 w266 w271 w275 w279 _ w285 w290 w294 w298 w302 _ _] -> w193
              tunnel: w191 -> [_ w203 _ _ _ _ _ _ _ _ _ _ _ _]
              event Timeout {
                n51 = event-data() -> ()  [unwired: 1 in, 3 out]
              }
              event "Test optotype": Mouse Wheel {
                n52 = event-data() -> ("Delta"=w202:i32)  [unwired: 1 in, 1 out]
                n53 = case shown="False" "IR refraction SM" {
                  tunnel: [0 1] -> w211
                  frame False {
                  }
                  frame True {
                  }
                }
                n54 = case shown="False" "VIS refraction SM" {
                  tunnel: [0 2] -> w210
                  frame False {
                  }
                  frame True {
                  }
                }
                n55 = case shown="False" "FIX refraction SM" {
                  tunnel: [0 3] -> w209
                  frame False {
                  }
                  frame True {
                  }
                }
                n56 = case shown="False" "IR brightness" {
                  tunnel: [0 4] -> w208
                  frame False {
                  }
                  frame True {
                  }
                }
                n57 = case shown="False" "VIS brightness" {
                  tunnel: [0 5] -> w207
                  frame False {
                  }
                  frame True {
                  }
                }
                n58 = Compound Arithmetic op=ADD(w211, w210, w209, w208, w207) -> (w206:i32)
                n59 = Sign(1:w202) -> (0:w201:i32)
                n60 = To Single Precision Float(number=w201) -> (single precision float=w200:sgl)
                n61 = case shown="5" w206 {
                  tunnel: w205 -> [_ w224 w230 w237 w244 w251]
                  tunnel: [errorcluster {"status"=FALSE, "code"=0, "source"=""} ("error out") w223 w231 w238 w245 w252] -> w204
                  tunnel: w203 -> [_ w222 w228 w235 w242 w249]
                  tunnel: w200 -> [_ w219 w226 w232 w241 w246]
                  frame 0, Default {
                  }
                  frame 1 {
                    n62 = Multiply(x="IR ref SM step [mm]", y=w219) -> (x*y=w221:sgl)
                    n63 = call "LensMotorsS3_move.vi"("error in (no error)"=w222, "delta"=w221, "channel"=w224) -> ("error out"=w223:errorcluster)  [unwired: 8 in]
                  }
                  frame 2 {
                    n64 = Multiply(x="VIS ref SM step [mm]", y=w226) -> (x*y=w225:sgl)
                    n65 = call "LensMotors_move.vi"("modIdTag"="S1", "error in (no error)"=w228, "delta"=w225, "channel"=w230) -> ("error out"=w231:errorcluster)  [unwired: 7 in]
                  }
                  frame 3 {
                    n66 = Multiply(x="FIX ref SM step [mm]", y=w232) -> (x*y=w234:sgl)
                    n67 = call "LensMotors_move.vi"("modIdTag"="S2", "error in (no error)"=w235, "delta"=w234, "channel"=w237) -> ("error out"=w238:errorcluster)  [unwired: 7 in]
                  }
                  frame 4 {
                    n68 = Multiply(x="IR br SM step [deg]", y=w241) -> (x*y=w239:sgl)
                    n69 = call "GF_MOVE.vi"("modIdTag"="F1", "error in (no error)"=w242, "delta"=w239, "channel"=w244) -> ("error out"=w245:errorcluster)  [unwired: 7 in]
                  }
                  frame 5 {
                    n70 = Multiply(x="VIS br SM step [deg]", y=w246) -> (x*y=w247:sgl)
                    n71 = call "GF_MOVE.vi"("modIdTag"="F2", "error in (no error)"=w249, "delta"=w247, "channel"=w251) -> ("error out"=w252:errorcluster)  [unwired: 7 in]
                  }
                }
              }
              event "IR shutter": Value Change {
                w263 = 1 items=["ServoUnspecified", "ServoCh1", "ServoCh2", "ServoBoth"] ("servo")
                n72 = event-data() -> ()  [unwired: 1 in, 2 out]
                n73 = call "shutter.vi"("servo"=w263, "Status"="IR shutter", "channel"=w265) -> ("error out"=w266:errorcluster)  [unwired: 8 in]
              }
              event "VIS shutter": Value Change {
                w269 = 2 items=["ServoUnspecified", "ServoCh1", "ServoCh2", "ServoBoth"] ("servo")
                n74 = event-data() -> ()  [unwired: 1 in, 2 out]
                n75 = call "shutter.vi"("servo"=w269, "Status"="VIS shutter", "channel"=w272) -> ("error out"=w271:errorcluster)  [unwired: 8 in]
              }
              event "Illuminator OFF": Value Change {
                n76 = event-data() -> ()  [unwired: 1 in, 2 out]
                n77 = call "ILL_ON-OFF.vi"("Boolean"="Illuminator OFF", "channel"=w274) -> ("error out"=w275:errorcluster)  [unwired: 9 in]
              }
              event "FIX OFF": Value Change {
                n78 = event-data() -> ()  [unwired: 1 in, 2 out]
                n79 = call "FIX_ON-OFF.vi"("Boolean"="FIX OFF", "channel"=w278) -> ("error out"=w279:errorcluster)  [unwired: 9 in]
              }
              event "OK Button 2": Value Change {
                n80 = event-data() -> ()  [unwired: 1 in, 2 out]
              }
              event "IR SM GTP": Value Change {
                n81 = event-data() -> ()  [unwired: 1 in, 2 out]
                n82 = call "LensMotors_go_to_position.vi"("modIdTag"="S3", "position"="IR SM GoToPos", "channel"=w286) -> ("error out"=w285:errorcluster)  [unwired: 8 in]
              }
              event "VIS SM GTP": Value Change {
                n83 = event-data() -> ()  [unwired: 1 in, 2 out]
                n84 = call "LensMotors_go_to_position.vi"("modIdTag"="S1", "position"="VIS SM GoToPos", "channel"=w289) -> ("error out"=w290:errorcluster)  [unwired: 8 in]
              }
              event "FIX SM GTP": Value Change {
                n85 = event-data() -> ()  [unwired: 1 in, 2 out]
                n86 = call "LensMotors_go_to_position.vi"("modIdTag"="S2", "position"="FIX SM GoToPos", "channel"=w293) -> ("error out"=w294:errorcluster)  [unwired: 8 in]
              }
              event "IR SM GTP": Value Change {
                n87 = event-data() -> ()  [unwired: 1 in, 2 out]
                n88 = call "GF_go_to_position.vi"("modIdTag"="F1", "position"="IR GF GoToPos", "channel"=w297) -> ("error out"=w298:errorcluster)  [unwired: 8 in]
              }
              event "VIS SM GTP": Value Change {
                n89 = event-data() -> ()  [unwired: 1 in, 2 out]
                n90 = call "GF_go_to_position.vi"("modIdTag"="F2", "position"="VIS GF GoToPos", "channel"=w301) -> ("error out"=w302:errorcluster)  [unwired: 8 in]
              }
              event "Select test optotype": Value Change {
                n91 = event-data() -> ()  [unwired: 1 in, 6 out]
              }
              event "Hide optotype": Value Change {
                n92 = event-data() -> ()  [unwired: 1 in, 6 out]
              }
            }
            n93 = Compound Arithmetic op=OR(w193, w194) -> (w196:bool)
          }
          frame "Set power" {
            # "Set the specified power value"
            n94 = local read "Set Max Power [W]"() -> (w320:dbl)
            n95 = Equal To 0?(x="Set power [W]") -> (x = 0?=w323:bool)
            n96 = Select(t=1e-06, s=w323, f="Set power [W]") -> (s? t:f=w319:dbl)
            n97 = Less Or Equal?(x=w319, y=w320) -> (x <= y?=w321:bool)
            n98 = local read "Set Min Power [W]"() -> (w311:dbl)
            n99 = Select(t=w319, s=w321, f=w320) -> (s? t:f=w312:dbl)
            n100 = local read "Power Value"() -> (w309:dbl)
            n101 = Greater Or Equal?(x=w312, y=w311) -> (x >= y?=w310:bool)
            n102 = Select(t=w312, s=w310, f=w311) -> (s? t:f=w308:dbl)
            n103 = Subtract(x=w309, y=w308) -> (x-y=w318:dbl)
            n104 = Absolute Value(x=w318) -> (abs(x)=w317:dbl)
            n105 = Multiply(x=w308, y=0.05) -> (x*y=w316:dbl)
            n106 = Less Or Equal?(x=w317, y=w316) -> (x <= y?=w315:bool)
            n107 = case shown="False" w315 {
              tunnel: [State_2."Set power" ("Enum") State_2."Wait for event" ("Enum")] -> w313
              tunnel: w309 -> [w339 _]
              tunnel: w308 -> [w338 _]
              tunnel: [w327 errorcluster {"status"=FALSE, "code"=0, "source"=""} ("error out")] -> w307
              tunnel: w306 -> [w328 _]
              frame False {
                n108 = call "Calculate_position.vi"("P(theta)"=w338, "P0"=w339) -> ("theta"=w337:dbl)  [unwired: 9 in]
                n109 = Wait (ms)(milliseconds to wait=u32 250) -> ()  [unwired: 1 out]
                n110 = To Single Precision Float(number=w337) -> (single precision float=w334:sgl)
                n111 = case shown="False" "Stimulus" {
                  tunnel: ["F1" "F2"] -> w329
                  frame False {
                  }
                  frame True {
                  }
                }
                n112 = call "GF_status.vi"("modIdTag"=w329, "channel"=w328) -> ("CurrPosition"=w333:sgl)  [unwired: 6 in, 3 out]
                n113 = Add(x=w334, y=w333) -> (x+y=w332:sgl)
                n114 = Quotient & Remainder(x=w332, y=sgl 360.0) -> (x-y*floor(x/y)=w330:sgl)  [unwired: 1 out]
                n115 = call "GF_go_to_position.vi"("modIdTag"=w329, "position"=w330, "channel"=w328) -> ("error out"=w327:errorcluster)  [unwired: 8 in]
              }
              frame True {
              }
            }
            n116 = Compound Arithmetic op=OR(w307, w324) -> (w325:bool)
          }
          frame "Update optotype" {
            w360 = 10123 items=["Finite Samples"=10178, "Continuous Samples"=10123, "Hardware Timed Single Point"=12522] ("sample mode")
            # "Update optotype"
            n117 = case shown="False" "Hide optotype" {
              tunnel: [w370 w407] -> w367
              tunnel: [w369 w405] -> w355
              tunnel: [w368 w406] -> w354
              frame False {
                n118 = case shown="0, Default" "Select test optotype" {
                  tunnel: "Size [V]" -> [w377 w381 w386 w389 _ _]
                  tunnel: [w376 w380 w385 w390 w395 w401] -> w368
                  tunnel: [w378 w379 w384 w392 w396 w400] -> w369
                  tunnel: [w375 w382 w383 w391 w397 w399] -> w370
                  tunnel: "X position" -> [_ _ _ w388 w394 w402]
                  tunnel: "Y position" -> [_ _ _ w387 w393 w398]
                  frame 0, Default {
                    n119 = call "Circle.vi"("Min/Max Voltage"=w377) -> ("Rate"=w376:dbl, "Scanners trajectories"=w378:dbl[][], "XY Graph"=w375:cluster{"sine wave":dbl[], "sine wave":dbl[]})  [unwired: 7 in]
                  }
                  frame 1 {
                    n120 = call "Cross.vi"("Min/Max Voltage"=w381) -> ("Rate"=w380:dbl, "Scanners trajectories"=w379:dbl[][], "XY Graph"=w382:cluster{dbl[], "Ramp Pattern":dbl[]})  [unwired: 8 in]
                  }
                  frame 2 {
                    n121 = call "Square.vi"("Min/Max Voltage"=w386) -> ("Rate"=w385:dbl, "Waveform Graph"=w384:dbl[][], "XY Graph"=w383:cluster{"Y":dbl[], "X":dbl[]})  [unwired: 8 in]
                  }
                  frame 3 {
                    n122 = call "Circle_flicker.vi"("shiftY"=w387, "shiftX"=w388, "Min&Max Voltage"=w389) -> ("Rate"=w390:dbl, "Scanners trajectories"=w392:dbl[][], "XY Graph"=w391:cluster{"sine wave":dbl[], "sine wave":dbl[]})  [unwired: 6 in]
                  }
                  frame 4 {
                    n123 = call "Beam.vi"("shiftY"=w393, "shiftX"=w394) -> ("Rate"=w395:dbl, "Scanners trajectories"=w396:dbl[][], "XY Graph"=w397:cluster{"sine wave":dbl[], "sine wave":dbl[]})  [unwired: 7 in]
                  }
                  frame 5 {
                    n124 = call "Beam_flicker_for_perimetry.vi"("shiftY"=w398, "shiftX"=w402) -> ("Rate"=w401:dbl, "Scanners trajectories"=w400:dbl[][], "XY Graph"=w399:cluster{dbl[], dbl[]})  [unwired: 7 in]
                  }
                }
              }
              frame True {
                n125 = call "Beam.vi"("shiftY"=4.0, "shiftX"=0.0) -> ("Rate"=w406:dbl, "Scanners trajectories"=w405:dbl[][], "XY Graph"=w407:cluster{"sine wave":dbl[], "sine wave":dbl[]})  [unwired: 7 in]
              }
            }
            "Test optotype" <- w367
            n126 = call <vilib>:"DAQmx Stop Task.vi"("task/channels in"=w352, "error in"=w351) -> ("task out"=w359:refnum<k21>, "error out"=w358:errorcluster)  [unwired: 12 in]
            n127 = call <vilib>:"DAQmx Is Task Done.vi"("task/channels in"=w359, "error in"=w358) -> ("task out"=w357:refnum<k21>, "error out"=w356:errorcluster)  [unwired: 11 in, 1 out]
            n128 = call-poly <vilib>:"DAQmx Timing.vi"("task/channels in"=w357, "sample mode"=w360, "rate"=w354, "error in"=w356) -> ("task out"=w366:refnum<k21>, "error out"=w361:errorcluster)  [unwired: 10 in]
            n129 = call-poly <vilib>:"DAQmx Write.vi"("task/channels in"=w366, "data"=w355, "error in"=w361) -> ("task out"=w365:refnum<k21>, "error out"=w363:errorcluster)  [unwired: 10 in, 1 out]
            n130 = call <vilib>:"DAQmx Start Task.vi"("task/channels in"=w365, "error in"=w363) -> ("task out"=w364:refnum<k21>, "error out"=w362:errorcluster)  [unwired: 12 in]
            n131 = call <vilib>:"DAQmx Is Task Done.vi"("task/channels in"=w364, "error in"=w362) -> ("task out"=w350:refnum<k21>, "error out"=w348:errorcluster)  [unwired: 11 in, 1 out]
            n132 = Compound Arithmetic op=OR(FALSE, w348) -> (w347:bool)
          }
        }
      }
      frame "Measurement" {
        n133 = case shown="\"Yes_2\"" w414 {
          tunnel: w422 -> [w445 w491 w517 w548 w566 w592 w629 w662 w706 w796 w842 w886 w935 w955 w978]
          tunnel: [w445 w491 w517 w548 w566 w592 w629 w662 w706 w795 w841 w885 w934 w955 w978] -> w420
          tunnel: [FALSE w490 FALSE FALSE ("status") FALSE ("status") w571 w616 FALSE w704 w798 FALSE w888 FALSE FALSE ("Is SM error occurred?") TRUE ("Is SM error occurred?")] -> w426
          tunnel: w428 -> [w437 w494 w523 w541 w559 w589 w626 w641 w705 w784 w830 w876 w925 w958 w971]
          tunnel: w427 -> [w436 w458 w512 w540 w558 w588 w625 w640 w700 w760 w815 w854 w912 w957 w970]
          tunnel: [w442 w494 w523 w543 w561 w589 w626 w658 w705 w784 w830 w876 w925 w958 w969] -> w419
          tunnel: [w441 w458 w512 w542 w560 w588 w625 w655 w700 w759 w815 w853 w912 w957 w963] -> w418
          tunnel: w425 -> [w444 w493 w522 w550 w568 w591 w628 _ w702 _ _ _ _ w956 w977]
          tunnel: [w444 w493 w522 w550 w568 w591 w628 0 w701 0 0 0 0 w956 w977] -> w424
          tunnel: [w443 w492 w518 w549 w567 w590 w627 w647 w699 w794 w840 w873 w922 w954 w976] -> w423
          tunnel: w421 -> [w443 w492 w518 w549 w567 w590 w627 w647 w699 w785 w831 w872 w921 w954 w976]
          tunnel: [w432 w485 w513 w537 w555 w577 w621 w634 w694 w768 w823 w863 w919 w953 w966] -> w416
          tunnel: w415 -> [w432 _ _ w537 w555 w577 w621 w634 w694 w768 w823 w863 w919 w953 w966]
          tunnel: [State."Idle_1" State."Set_power_2" w510 State."Set_power_2" w553 w576 State."Show optotype" State."Wait for event" w693 State."Random brightness" State."Hide optotype_1" State."Random brightness" State."Hide optotype_1" w951 State."Exit"] -> w413
          tunnel: w412 -> [w430 w462 w507 w535 w554 w574 w619 w632 w692 w762 w822 w856 _ w950 w964]
          tunnel: [w430 w462 w507 w535 w554 w574 w619 w632 w692 w762 w822 w856 TRUE w950 w964] -> w411
          tunnel: w410 -> [_ _ _ _ _ _ _ _ _ _ _ _ w909 _ _]
          tunnel: w409 -> [w429 w459 w506 w534 w552 w573 w618 w631 w691 w761 w814 w855 w910 w948 w961]
          tunnel: [w429 w459 w506 w534 w552 w573 w618 w631 w691 w761 w814 w855 w910 w948 w961] -> w408
          frame "Initialize", Default {
            w433 = 0.0 ("X coordinate")
            n134 = call <vilib>:"DAQmx Stop Task.vi"("task/channels in"=w437, "error in"=w436) -> ("task out"=w440:refnum<k21>, "error out"=w439:errorcluster)  [unwired: 12 in]
            n135 = call <vilib>:"DAQmx Is Task Done.vi"("task/channels in"=w440, "error in"=w439) -> ("task out"=w438:refnum<k21>, "error out"=w435:errorcluster)  [unwired: 11 in, 1 out]
            n136 = call "Hide_scanners.vi"("error in"=w435, "Y coordinate"=w433, "X coordinate"=w433, "task/channels in"=w438) -> ("error out"=w441:errorcluster, "task out"=w442:refnum<k21>)  [unwired: 6 in]
          }
          frame "Idle_2" {
            # "Wait for the start of the measurement (Start measurement button)\n\nIf you press this button, tables (XY coordinates, threshold values etc) will be created"
            n137 = Increment(x="Number of points M-2") -> (x+1=w452:i32)
            n138 = To Single Precision Float(number=w452) -> (single precision float=w475:sgl)
            n139 = Divide(x="Number of points M-2", y=2.0) -> (x/y=w449:dbl)
            n140 = Divide(x="Investigated brightness range [dB]", y=w475) -> (x/y=w457:sgl)
            n141 = local read "Init filter position"() -> (w453:sgl)
            n142 = Round Toward -Infinity(1:w449) -> (0:w448:dbl)
            n143 = Negate(x=w448) -> (-x=w447:dbl)
            n144 = Add(x="Number of points M-2", y=2) -> (x+y=w461:i32)
            n145 = Multiply(x=w457, y=sgl 8.6) -> (x*y=w456:sgl)
            n146 = To Single Precision Float(number=w447) -> (single precision float=w446:sgl)
            n147 = for {
              N: w461 -> [_]
              tunnel: [i32[] [0, 0]] -> w478 mode=indexing
              tunnel: [FALSE] -> w476 mode=indexing
            }
            "Found?" <- w476
            "C brightness" <- w476
            "Answers" <- w478
            n148 = for {
              N: "Number of points M-2" -> [_]
              tunnel: w456 -> [w502]
              tunnel: [w501] -> w471 mode=indexing
              tunnel: [w500] -> w463
              tunnel: w453 -> [w499]
              tunnel: w446 -> [w497]
              i -> [w500]
              n149 = To Single Precision Float(number=w500) -> (single precision float=w498:sgl)
              n150 = Add(x=w497, y=w498) -> (x+y=w496:sgl)
              n151 = Multiply(x=w496, y=w502) -> (x*y=w495:sgl)
              n152 = Add(x=w499, y=w495) -> (x+y=w501:sgl)
            }
            n153 = Get Date/Time In Seconds() -> (seconds since 1Jan1904=→"Measur. start time":timestamp)
            n154 = Multiply(x="Number of trials k", y=w461) -> (x*y=w473:i32)
            n155 = To Double Precision Float(number=w473) -> (double precision float=w472:dbl)
            n156 = To Double Precision Float(number=w461) -> (double precision float=w460:dbl)
            n157 = Index Array(array=w471, index=w463) -> (element=w466:sgl)
            n158 = Index Array(array=w471, index=0) -> (element=w469:sgl)
            n159 = Add(x=w466, y=sgl 25.8) -> (x+y=w465:sgl)
            n160 = Subtract(x=w469, y=sgl 25.8) -> (x-y=w468:sgl)
            n161 = property on="Progress - found locations" class="Slide (strict)"("Scale.Maximum"=w472, "Scale.Minimum"=0.0 ("Data Entry Limits:Minimum"), "Increment"=1.0 ("Data Entry Limits:Increment")) -> (error out=w488:errorcluster)  [unwired: 2 in, 1 out]
            n162 = Build Array (concatenate)(w468, w471, w465) -> (→"Filter positions [deg]":sgl[])
            n163 = Divide(x=w460, y=2.0) -> (x/y=w487:dbl)
            n164 = Round To Nearest(number=w487) -> (nearest integer value=w486:dbl)
            n165 = To Long Integer(number=w486) -> (32bit integer=w485:i32)
            n166 = Compound Arithmetic op=OR(w488, FALSE) -> (w490:bool)
          }
          frame "Random brightness" {
            # "Select the power level\n\nAvoid to choose the levels for which the threshold is found\n\nUpdate C brightness (current brightness) table values\n\nIf  all thresholds are found, go to exit"
            n167 = local read "Number of points M-2"() -> (w511:i32)
            n168 = Increment(x=w511) -> (x+1=w509:i32)
            n169 = Random Number (0-1)() -> (number: 0 to 1=w521:dbl)
            n170 = To Double Precision Float(number=w509) -> (double precision float=w508:dbl)
            n171 = Multiply(x=w521, y=w508) -> (x*y=w520:dbl)
            n172 = Round To Nearest(number=w520) -> (nearest integer value=w519:dbl)
            n173 = To Long Integer(number=w519) -> (32bit integer=w513:i32)
            n174 = local read "Found?"() -> (w514:bool[])
            n175 = Index Array(array=w514, index=w513) -> (element=w515:bool)
            n176 = And Array Elements(Boolean array=w514) -> (logical AND=w516:bool)
            n177 = case shown="True" w515 {
              tunnel: [State."Hide optotype_2" w530] -> w510
              tunnel: w516 -> [_ w529]
              tunnel: w513 -> [w525 _]
              frame False {
                n178 = local read "C brightness"() -> (w527:bool[])
                n179 = Replace Array Subset(array=w527, new element=TRUE ("new element/subarray"), index=w525) -> (w528:bool[])
                n180 = local write "C brightness"(w528) -> ()
              }
              frame True {
                n181 = case shown="False" w529 {
                  tunnel: [State."Random brightness" ("Enum") State."Exit" ("Enum")] -> w530
                  frame False {
                  }
                  frame True {
                  }
                }
              }
            }
          }
          frame "Hide optotype_2" {
            n182 = call <vilib>:"DAQmx Stop Task.vi"("task/channels in"=w541, "error in"=w540) -> ("task out"=w547:refnum<k21>, "error out"=w546:errorcluster)  [unwired: 12 in]
            n183 = call <vilib>:"DAQmx Is Task Done.vi"("task/channels in"=w547, "error in"=w546) -> ("task out"=w545:refnum<k21>, "error out"=w544:errorcluster)  [unwired: 11 in, 1 out]
            n184 = local read "X position"() -> (w539:dbl)
            n185 = local read "Y position"() -> (w538:dbl)
            n186 = call "Hide_scanners.vi"("error in"=w544, "Y coordinate"=w538, "X coordinate"=w539, "task/channels in"=w545) -> ("error out"=w542:errorcluster, "task out"=w543:refnum<k21>)  [unwired: 6 in]
          }
          frame "Hide optotype_1" {
            n187 = case shown="False" w554 {
              tunnel: [State."Set power_1" State."Idle_2"] -> w553
              frame False {
              }
              frame True {
              }
            }
            n188 = call <vilib>:"DAQmx Stop Task.vi"("task/channels in"=w559, "error in"=w558) -> ("task out"=w565:refnum<k21>, "error out"=w564:errorcluster)  [unwired: 12 in]
            n189 = call <vilib>:"DAQmx Is Task Done.vi"("task/channels in"=w565, "error in"=w564) -> ("task out"=w563:refnum<k21>, "error out"=w562:errorcluster)  [unwired: 11 in, 1 out]
            n190 = local read "X position"() -> (w557:dbl)
            n191 = local read "Y position"() -> (w556:dbl)
            n192 = call "Hide_scanners.vi"("error in"=w562, "Y coordinate"=w556, "X coordinate"=w557, "task/channels in"=w563) -> ("error out"=w560:errorcluster, "task out"=w561:refnum<k21>)  [unwired: 6 in]
          }
          frame "Set power_1" {
            n193 = Equal?(x="Init power level [W]", y=0.0) -> (x = y?=w581:bool)
            n194 = local read "Power Value"() -> (w578:dbl)
            n195 = Select(t=1e-06, s=w581, f="Init power level [W]") -> (s? t:f=w579:dbl)
            n196 = Subtract(x=w578, y=w579) -> (x-y=w587:dbl)
            n197 = Absolute Value(x=w587) -> (abs(x)=w586:dbl)
            n198 = Multiply(x=w579, y=0.05) -> (x*y=w585:dbl)
            n199 = Less Or Equal?(x=w586, y=w585) -> (x <= y?=w583:bool)
            n200 = case shown="False" w583 {
              tunnel: [State."Set power_1" State."Show optotype"] -> w576
              tunnel: w579 -> [w604 _]
              tunnel: w578 -> [w605 _]
              tunnel: w573 -> [w595 _]
              tunnel: [w598 errorcluster {"status"=FALSE, "code"=0, "source"=""} ("error out")] -> w572
              frame False {
                n201 = call "Calculate_position.vi"("P(theta)"=w604, "P0"=w605) -> ("theta"=w606:dbl)  [unwired: 9 in]
                n202 = Wait (ms)(milliseconds to wait=u32 250) -> ()  [unwired: 1 out]
                n203 = To Single Precision Float(number=w606) -> (single precision float=w597:sgl)
                n204 = case shown="True" "Filter" {
                  tunnel: ["F1" "F2"] -> w596
                  frame False {
                  }
                  frame True {
                  }
                }
                n205 = call "GF_status.vi"("modIdTag"=w596, "channel"=w595) -> ("error out"=w594:errorcluster, "CurrPosition"=w602:sgl)  [unwired: 6 in, 2 out]
                n206 = Add(x=w597, y=w602) -> (x+y=w601:sgl)
                n207 = Quotient & Remainder(x=w601, y=sgl 360.0) -> (x-y*floor(x/y)=w599:sgl)  [unwired: 1 out]
                n208 = call "GF_go_to_position.vi"("modIdTag"=w596, "error in (no error)"=w594, "position"=w599, "channel"=w595) -> ("error out"=w598:errorcluster)  [unwired: 7 in]
              }
              frame True {
              }
            }
            n209 = Compound Arithmetic op=OR(w572) -> (w571:bool)
          }
          frame "Set_power_2" {
            n210 = local read "Filter positions [deg]"() -> (w614:sgl[])
            n211 = Array Subset(array=w614, index=w621, length=1) -> (w622:sgl[])
            n212 = Array To Cluster(array=w622) -> (cluster=w623:cluster{"[0]":sgl})
            n213 = Unbundle(w623) -> ("[0]"=w613:sgl)
            n214 = Wait (ms)(milliseconds to wait=u32 250) -> ()  [unwired: 1 out]
            n215 = call "GF_go_to_position.vi"("modIdTag"="F1", "position"=w613, "channel"=w618) -> ("error out"=w617:errorcluster)  [unwired: 8 in]
            n216 = Compound Arithmetic op=AND(w617) -> (w616:bool)
          }
          frame "Show optotype" {
            w648 = 10123 items=["Finite Samples"=10178, "Continuous Samples"=10123, "Hardware Timed Single Point"=12522] ("sample mode")
            n217 = local read "X position"() -> (w636:dbl)
            n218 = local read "Y position"() -> (w635:dbl)
            n219 = call <vilib>:"DAQmx Stop Task.vi"("task/channels in"=w641, "error in"=w640) -> ("task out"=w646:refnum<k21>, "error out"=w645:errorcluster)  [unwired: 12 in]
            n220 = call <vilib>:"Beep.vi"("use system alert? (T)"=FALSE, "duration (msec)"=u32 300, "frequency (Hz)"=u32 1050) -> ()  [unwired: 9 in]
            n221 = call <vilib>:"DAQmx Is Task Done.vi"("task/channels in"=w646, "error in"=w645) -> ("task out"=w644:refnum<k21>, "error out"=w643:errorcluster)  [unwired: 11 in, 1 out]
            n222 = case shown="5" "Select optotype" {
              tunnel: "Min/Max Voltage" -> [w665 w669 w674 w677 _ _]
              tunnel: [w664 w668 w673 w680 w683 w690] -> w657
              tunnel: [w666 w667 w672 w679 w684 w689] -> w656
              tunnel: [w663 w670 w671 w678 w685 w688] -> w659
              tunnel: w636 -> [_ _ _ w676 w682 w687]
              tunnel: w635 -> [_ _ _ w675 w681 w686]
              frame 0, Default {
                n223 = call "Circle.vi"("Min/Max Voltage"=w665) -> ("Rate"=w664:dbl, "Scanners trajectories"=w666:dbl[][], "XY Graph"=w663:cluster{"sine wave":dbl[], "sine wave":dbl[]})  [unwired: 7 in]
              }
              frame 1 {
                n224 = call "Cross.vi"("Min/Max Voltage"=w669) -> ("Rate"=w668:dbl, "Scanners trajectories"=w667:dbl[][], "XY Graph"=w670:cluster{dbl[], "Ramp Pattern":dbl[]})  [unwired: 8 in]
              }
              frame 2 {
                n225 = call "Square.vi"("Min/Max Voltage"=w674) -> ("Rate"=w673:dbl, "Waveform Graph"=w672:dbl[][], "XY Graph"=w671:cluster{"Y":dbl[], "X":dbl[]})  [unwired: 8 in]
              }
              frame 3 {
                n226 = call "Circle_flicker_for_perimetry.vi"("shiftY"=w675, "shiftX"=w676, "Min&Max Voltage"=w677) -> ("Rate"=w680:dbl, "Scanners trajectories"=w679:dbl[][], "XY Graph"=w678:cluster{"sine wave":dbl[], "sine wave":dbl[]})  [unwired: 6 in]
              }
              frame 4 {
                n227 = call "Beam.vi"("shiftY"=w681, "shiftX"=w682) -> ("Rate"=w683:dbl, "Scanners trajectories"=w684:dbl[][], "XY Graph"=w685:cluster{"sine wave":dbl[], "sine wave":dbl[]})  [unwired: 7 in]
              }
              frame 5 {
                n228 = call "Beam_flicker_for_perimetry.vi"("shiftY"=w686, "shiftX"=w687) -> ("Rate"=w690:dbl, "Scanners trajectories"=w689:dbl[][], "XY Graph"=w688:cluster{dbl[], dbl[]})  [unwired: 7 in]
              }
            }
            "XY Graph" <- w659
            "Rate" <- w657
            n229 = call-poly <vilib>:"DAQmx Timing.vi"("task/channels in"=w644, "sample mode"=w648, "rate"=w657, "error in"=w643) -> ("task out"=w654:refnum<k21>, "error out"=w649:errorcluster)  [unwired: 10 in]
            n230 = call-poly <vilib>:"DAQmx Write.vi"("task/channels in"=w654, "data"=w656, "error in"=w649) -> ("task out"=w653:refnum<k21>, "error out"=w651:errorcluster)  [unwired: 10 in, 1 out]
            n231 = call <vilib>:"DAQmx Start Task.vi"("task/channels in"=w653, "error in"=w651) -> ("task out"=w652:refnum<k21>, "error out"=w650:errorcluster)  [unwired: 12 in]
            n232 = call <vilib>:"DAQmx Is Task Done.vi"("task/channels in"=w652, "error in"=w650) -> ("task out"=w658:refnum<k21>, "error out"=w655:errorcluster)  [unwired: 11 in, 1 out]
          }
          frame "Wait for event" {
            # "Wait for event\n\n1. If timeout and all threshold found - go to \"Exit\" \n2. If timeout but some thresholds are not found  or NO button=true - go to \"No\".\n                             After 10 iterations sound signal appears\n3. If \"Patient button\" or YES button= true -> go to \"Yes\""
            # "Response time: 1.0 sec"
            n233 = local read "Patient button"() -> (w695:bool)
            n234 = case shown="True" "Pause" {
              frame False {
              }
              frame True {
                n235 = while {
                  stop <- w709 continue-if-true
                  n236 = local read "Pause"() -> (w709:bool)
                  n237 = Wait (ms)(milliseconds to wait=u32 100) -> ()  [unwired: 1 out]
                }
              }
            }
            n238 = case shown="True" w695 {
              selector: w695 -> [_ w710]
              frame False {
              }
              frame True {
                n239 = property on="Patient button" class="Bool (strict)"("Val(Sgnl)"=w710) -> ()  [unwired: 2 in, 2 out]
              }
            }
            n240 = local read "Found?"() -> (w696:bool[])
            n241 = And Array Elements(Boolean array=w696) -> (logical AND=w698:bool)
            n242 = event shown="[3] \"Patient button\": Value Change" {
              selector: _ -> [_ _ _ _]
              dyn-events: _ -> [_ _ _ _]
              timeout: 100 -> [_ _ _ _]
              tunnel: [w715 w732 w741 w751] -> w693
              tunnel: w702 -> [w716 w734 w743 w752]
              tunnel: [w714 w734 w743 w752] -> w701
              tunnel: w698 -> [w712 _ _ _]
              tunnel: w692 -> [w711 w731 w740 w749]
              event Timeout {
                n243 = event-data() -> ()  [unwired: 1 in, 1 out]
                n244 = And(x=w712, y=w711) -> (x .and. y?=w713:bool)
                n245 = case shown="False" w713 {
                  tunnel: w716 -> [w718 w722]
                  tunnel: [State."Exit" w721] -> w715
                  tunnel: [w718 w720] -> w714
                  tunnel: w711 -> [_ w719]
                  frame True {
                  }
                  frame False {
                    n246 = case shown="10" w722 {
                      selector: w722 -> [w725 _]
                      tunnel: [State."Wait for event" w727] -> w721
                      tunnel: [w723 0] -> w720
                      tunnel: w719 -> [_ w726]
                      frame Default {
                        n247 = Increment(x=w725) -> (x+1=w723:i32)
                      }
                      frame 10 {
                        n248 = case shown="True" w726 {
                          tunnel: [State."No_1" State."No_2"] -> w727
                          frame False {
                          }
                          frame True {
                          }
                        }
                      }
                    }
                  }
                }
              }
              event "YES button": Value Change {
                n249 = event-data() -> ("NewVal"=w733:bool)  [unwired: 1 in]
                n250 = case shown="True" w733 {
                  tunnel: [State."Wait for event" w737] -> w732
                  tunnel: w731 -> [_ w736]
                  frame False {
                  }
                  frame True {
                    n251 = case shown="True" w736 {
                      tunnel: [State."Yes_1" State."Yes_2"] -> w737
                      frame False {
                      }
                      frame True {
                      }
                    }
                  }
                }
              }
              event "NO button": Value Change {
                n252 = event-data() -> ("NewVal"=w742:bool)  [unwired: 1 in]
                n253 = case shown="True" w742 {
                  tunnel: [State."Wait for event" w745] -> w741
                  tunnel: w740 -> [_ w746]
                  frame False {
                  }
                  frame True {
                    n254 = case shown="False" w746 {
                      tunnel: [State."No_1" State."No_2"] -> w745
                      frame False {
                      }
                      frame True {
                      }
                    }
                  }
                }
              }
              event "Patient button": Value Change {
                n255 = event-data() -> ("NewVal"=w750:bool)  [unwired: 1 in]
                n256 = case shown="True" w750 {
                  tunnel: [State."Wait for event" w754] -> w751
                  tunnel: w749 -> [_ w755]
                  frame False {
                  }
                  frame True {
                    n257 = property on="Patient button" class="Bool (strict)"("Value"=FALSE ("Patient button")) -> ()  [unwired: 2 in, 2 out]
                    n258 = case shown="False" w755 {
                      tunnel: [State."Yes_1" State."Yes_2"] -> w754
                      frame False {
                      }
                      frame True {
                      }
                    }
                  }
                }
              }
            }
            n259 = Compound Arithmetic op=OR(FALSE, w700) -> (w704:bool)
          }
          frame "Yes_2" {
            w770 = 1 ("length")
            n260 = disable-structure shown="Enabled" {
              disable-tunnel: [w804 w811] -> w787
              disable-tunnel: w768 -> [w803 w812]
              frame Disabled {
                n261 = case shown="0" w803 {
                  tunnel: ["C" "U" "D" "L" "R" "error"] -> w804
                  frame 0 {
                  }
                  frame 1 {
                  }
                  frame 2 {
                  }
                  frame 3 {
                  }
                  frame 4 {
                  }
                  frame 5, Default {
                  }
                }
              }
              frame Enabled {
                n262 = Number To Decimal String(number=w812) -> (decimal integer string=w811:string)  [unwired: 1 in]
              }
            }
            n263 = local read "Answers"() -> (w771:i32[][])
            n264 = local read "Measur. start time"() -> (w789:timestamp)
            n265 = Wait (ms)(milliseconds to wait=u32 1000) -> ()  [unwired: 1 out]
            n266 = Array Subset(array=w771, index (row)=w768, length (row)=w770, index (col)=0 ("index"), length (col)=w770) -> (w773:i32[][])
            n267 = local read "Power Value"() -> (w782:dbl)
            n268 = Get Date/Time In Seconds() -> (seconds since 1Jan1904=w792:timestamp)
            n269 = call <vilib>:"Beep.vi"("use system alert? (T)"=FALSE, "duration (msec)"=u32 50, "frequency (Hz)"=u32 1568) -> ()  [unwired: 9 in]
            n270 = Increment(x=w773) -> (x+1=w772:i32[][])
            n271 = Subtract(x=w792, y=w789) -> (x-y=w790:dbl)
            n272 = Replace Array Subset(array=w771, new element=w772, index (row)=w768, index (col)=0 ("disabled index (col)")) -> (w766:i32[][])
            n273 = local read "Number of trials k"() -> (w774:i32)
            n274 = property on="Progress - found locations" class="Slide (strict)"() -> (error out=w763:errorcluster, "Value"=w765:u8)  [unwired: 2 in, 1 out]
            n275 = Bundle("Power Value"=w782, w787, "Y", w790, "seconds since 1Jan1904"=w792) -> (w791:T6)  [unwired: 1 in]
            n276 = Build Cluster Array(w791) -> (w783:T7)
            n277 = Index Array(array=w766, index (row)=w768) -> (element=w777:i32[])  [unwired: 1 in]
            n278 = Increment(x=w765) -> (x+1=w764:u8)
            n279 = local write "Answers"(w766) -> ()
            n280 = Insert Into Array(array=w796, index=w785, new element=w783) -> (w795:T2)
            n281 = Add Array Elements(numeric array=w777) -> (sum=w776:i32)
            n282 = property on="Progress - found locations" class="Slide (strict)"(error in=w763, "Value"=w764) -> (error out=w759:errorcluster)  [unwired: 1 in, 1 out]
            n283 = Equal?(x=w776, y=w774) -> (x = y?=w775:bool)
            n284 = case shown="True" w775 {
              tunnel: w768 -> [_ w800]
              frame False {
              }
              frame True {
                n285 = local read "Found?"() -> (w802:bool[])
                n286 = Replace Array Subset(array=w802, new element=TRUE ("new element/subarray"), index=w800) -> (w801:bool[])
                n287 = local write "Found?"(w801) -> ()
              }
            }
            n288 = Increment(x=w785) -> (x+1=w794:i32)
            n289 = Compound Arithmetic op=OR(FALSE, w760, w759) -> (w798:bool)
          }
          frame "Yes_1" {
            n290 = disable-structure shown="Enabled" {
              disable-tunnel: [w844 w851] -> w833
              disable-tunnel: w823 -> [w843 w852]
              frame Disabled {
                n291 = case shown="0" w843 {
                  tunnel: ["C" "U" "D" "L" "R" "error"] -> w844
                  frame 0 {
                  }
                  frame 1 {
                  }
                  frame 2 {
                  }
                  frame 3 {
                  }
                  frame 4 {
                  }
                  frame 5, Default {
                  }
                }
              }
              frame Enabled {
                n292 = Number To Decimal String(number=w852) -> (decimal integer string=w851:string)  [unwired: 1 in]
              }
            }
            n293 = local read "Init power level [W]"() -> (w819:dbl)
            n294 = local read "Measur. start time"() -> (w835:timestamp)
            n295 = Wait (ms)(milliseconds to wait=u32 1000) -> ()  [unwired: 1 out]
            n296 = local read "Power Value"() -> (w828:dbl)
            n297 = Get Date/Time In Seconds() -> (seconds since 1Jan1904=w838:timestamp)
            n298 = call <vilib>:"Beep.vi"("use system alert? (T)"=FALSE, "duration (msec)"=u32 50, "frequency (Hz)"=u32 1568) -> ()  [unwired: 9 in]
            n299 = Multiply(x=0.1, y="Threshold finding step [dB]") -> (x*y=w817:dbl)
            n300 = Subtract(x=w838, y=w835) -> (x-y=w836:dbl)
            n301 = Power Of 10(x=w817) -> (10^x=w816:dbl)
            n302 = Bundle("Power Value"=w828, w833, "Y", w836, "seconds since 1Jan1904"=w838) -> (w837:T6)  [unwired: 1 in]
            n303 = Build Cluster Array(w837) -> (w829:T7)
            n304 = Insert Into Array(array=w842, index=w831, new element=w829) -> (w841:T2)
            n305 = Divide(x=w819, y=w816) -> (x/y=w818:dbl)
            n306 = local write "Init power level [W]"(w818) -> ()
            n307 = Increment(x=w831) -> (x+1=w840:i32)
          }
          frame "No_2" {
            w866 = 1 ("length")
            n308 = disable-structure shown="Enabled" {
              disable-tunnel: [w894 w902] -> w878
              disable-tunnel: w863 -> [w893 w901]
              frame Disabled {
                n309 = case shown="5, Default" w893 {
                  tunnel: ["C" "U" "D" "L" "R" "error"] -> w894
                  frame 0 {
                  }
                  frame 1 {
                  }
                  frame 2 {
                  }
                  frame 3 {
                  }
                  frame 4 {
                  }
                  frame 5, Default {
                  }
                }
              }
              frame Enabled {
                n310 = Number To Decimal String(number=w901) -> (decimal integer string=w902:string)  [unwired: 1 in]
              }
            }
            n311 = local read "Answers"() -> (w864:i32[][])
            n312 = Wait (ms)(milliseconds to wait=u32 1000) -> ()  [unwired: 1 out]
            n313 = local read "Measur. start time"() -> (w880:timestamp)
            n314 = Array Subset(array=w864, index (row)=w863, length (row)=w866, index (col)=w866, length (col)=w866) -> (w865:i32[][])
            n315 = local read "Power Value"() -> (w875:dbl)
            n316 = Get Date/Time In Seconds() -> (seconds since 1Jan1904=w883:timestamp)
            n317 = Increment(x=w865) -> (x+1=w861:i32[][])
            n318 = property on="Progress - found locations" class="Slide (strict)"() -> (error out=w859:errorcluster, "Value"=w858:u8)  [unwired: 2 in, 1 out]
            n319 = Replace Array Subset(array=w864, new element=w861, index (row)=w863, index (col)=1 ("disabled index (col)")) -> (w860:i32[][])
            n320 = Subtract(x=w883, y=w880) -> (x-y=w881:dbl)
            n321 = Increment(x=w858) -> (x+1=w857:u8)
            n322 = Bundle("Power Value"=w875, w878, "N", w881, "seconds since 1Jan1904"=w883) -> (w882:T6)  [unwired: 1 in]
            n323 = local read "Number of trials k"() -> (w868:i32)
            n324 = Build Cluster Array(w882) -> (w874:T7)
            n325 = Index Array(array=w860, index (row)=w863) -> (element=w870:i32[])  [unwired: 1 in]
            n326 = local write "Answers"(w860) -> ()
            n327 = Insert Into Array(array=w886, index=w872, new element=w874) -> (w885:T2)
            n328 = property on="Progress - found locations" class="Slide (strict)"(error in=w859, "Value"=w857) -> (error out=w853:errorcluster)  [unwired: 1 in, 1 out]
            n329 = Add Array Elements(numeric array=w870) -> (sum=w869:i32)
            n330 = Equal?(x=w869, y=w868) -> (x = y?=w867:bool)
            n331 = case shown="True" w867 {
              tunnel: w863 -> [_ w890]
              frame False {
              }
              frame True {
                n332 = local read "Found?"() -> (w892:bool[])
                n333 = Replace Array Subset(array=w892, new element=TRUE ("new element/subarray"), index=w890) -> (w891:bool[])
                n334 = local write "Found?"(w891) -> ()
              }
            }
            n335 = Increment(x=w872) -> (x+1=w873:i32)
            n336 = Compound Arithmetic op=OR(FALSE, w854, w853) -> (w888:bool)
          }
          frame "No_1" {
            # "Pause for a subject"
            n337 = disable-structure shown="Enabled" {
              disable-tunnel: [w939 w947] -> w927
              disable-tunnel: w919 -> [w938 w946]
              frame Disabled {
                n338 = case shown="5, Default" w938 {
                  tunnel: ["C" "U" "D" "L" "R" "error"] -> w939
                  frame 0 {
                  }
                  frame 1 {
                  }
                  frame 2 {
                  }
                  frame 3 {
                  }
                  frame 4 {
                  }
                  frame 5, Default {
                  }
                }
              }
              frame Enabled {
                n339 = Number To Decimal String(number=w946) -> (decimal integer string=w947:string)  [unwired: 1 in]
              }
            }
            n340 = local read "Filter"() -> (w908:bool)
            n341 = local read "Threshold finding step [dB]"() -> (w918:dbl)
            n342 = case shown="False" w908 {
              tunnel: ["F1" "F2"] -> w907
              frame False {
              }
              frame True {
              }
            }
            n343 = local read "Init power level [W]"() -> (w914:dbl)
            n344 = local read "Measur. start time"() -> (w929:timestamp)
            n345 = call "GF_status.vi"("modIdTag"=w907, "error in (no error)"=w909, "channel"=w910) -> ("CurrPosition"=w906:sgl)  [unwired: 5 in, 3 out]
            n346 = local read "Power Value"() -> (w924:dbl)
            n347 = Get Date/Time In Seconds() -> (seconds since 1Jan1904=w932:timestamp)
            n348 = Multiply(x=w918, y=0.05) -> (x*y=w916:dbl)
            n349 = Wait (ms)(milliseconds to wait=u32 1000) -> ()  [unwired: 1 out]
            n350 = Power Of 10(x=w916) -> (10^x=w905:dbl)
            n351 = Subtract(x=w932, y=w929) -> (x-y=w930:dbl)
            n352 = Bundle("Power Value"=w924, w927, "N", w930, "seconds since 1Jan1904"=w932) -> (w931:T6)  [unwired: 1 in]
            n353 = Multiply(x=w914, y=w905) -> (x*y=w915:dbl)
            n354 = To Single Precision Float(number=w905) -> (single precision float=w904:sgl)
            n355 = Build Cluster Array(w931) -> (w923:T7)
            n356 = local write "Init power level [W]"(w915) -> ()
            n357 = Insert Into Array(array=w935, index=w921, new element=w923) -> (w934:T2)
            n358 = Add(x=w906, y=w904) -> (x+y=→"Init filter position":sgl)
            n359 = Increment(x=w921) -> (x+1=w922:i32)
          }
          frame "Idle_1" {
            n360 = event shown="[0] Timeout" {
              selector: _ -> [_ _]
              dyn-events: _ -> [_ _]
              timeout: 100 -> [_ _]
              tunnel: [State."Idle_1" State."Set power_1"] -> w951
              event Timeout {
                n361 = event-data() -> ()  [unwired: 1 in, 3 out]
              }
              event "Start measurement": Value Change {
                n362 = event-data() -> ()  [unwired: 1 in, 6 out]
              }
            }
          }
          frame "Exit" {
            # "Hide scanners and exit the program"
            n363 = call <vilib>:"DAQmx Stop Task.vi"("task/channels in"=w971, "error in"=w970) -> ("task out"=w975:refnum<k21>, "error out"=w974:errorcluster)  [unwired: 12 in]
            n364 = call <vilib>:"DAQmx Is Task Done.vi"("task/channels in"=w975, "error in"=w974) -> ("task out"=w973:refnum<k21>, "error out"=w972:errorcluster)  [unwired: 11 in, 1 out]
            n365 = local read "Y position"() -> (w967:dbl)
            n366 = local read "X position"() -> (w968:dbl)
            n367 = call "Hide_scanners.vi"("error in"=w972, "Y coordinate"=w967, "X coordinate"=w968, "task/channels in"=w973) -> ("error out"=w963:errorcluster, "task out"=w969:refnum<k21>)  [unwired: 6 in]
          }
        }
      }
    }
    "Previous brightess" <- w157
    "Enum" <- w155
    n368 = property on="loop up cond." class="Bool (strict)"() -> (error out=w124:errorcluster, "Value"=w123:bool)  [unwired: 2 in, 1 out]
    n369 = Wait (ms)(milliseconds to wait=u32 3) -> ()  [unwired: 1 out]
    n370 = Compound Arithmetic op=OR(w174, w165, w124, w123) -> (w160:bool)
    "loop down cond." <- w160
    "Threshold found?" <- w154
  }
  n371 = while {
    tunnel: w23 -> [w1025]
    tunnel: w13 -> [w1018]
    tunnel: [w1016] -> w11
    tunnel: [w979] -> w31
    tunnel: w26 -> [w1028]
    tunnel: [w1026] -> w24
    tunnel: w21 -> [w1023]
    tunnel: [w1021] -> w19
    tunnel: [w980] -> w32
    tunnel: w15 -> [w1020]
    tunnel: [w1027] -> w25
    tunnel: w14 -> [w1019]
    tunnel: [w1017] -> w12
    tunnel: w22 -> [w1024]
    tunnel: [w1022] -> w20
    tunnel: w5 -> [w981]
    tunnel: w4 -> [w982]
    stop <- w1008 stop-if-true
    n372 = control-ref of="Pixel clock"() -> (w990:refnum<vi>)
    n373 = control-ref of="Frame rate"() -> (w989:refnum<vi>)
    n374 = control-ref of="Exposure time"() -> (w988:refnum<vi>)
    n375 = control-ref of="Gain"() -> (w987:refnum<vi>)
    n376 = call "TLPMX Measure Power.vi"("error in (no error)"=w982, "instrument handle"=w981) -> ("error out"=w979:errorcluster, "Power"=→"Power Value":dbl, "instrument handle out"=w980:refnum<visa-resource-name>)  [unwired: 7 in]
    n377 = call-poly <vilib>:"DAQmx Read.vi"("task/channels in"=w1019, "error in"=w1018) -> ("task out"=w1017:refnum<k21>, "data"=→"Patient button":bool, "error out"=w1016:errorcluster)  [unwired: 11 in]
    n378 = Bundle("Pixel clock"=w990, "Frame rate"=w989, "Exposure time"=w988, "Gain"=w987, "Auto gain"="Auto gain") -> (w985:T8)  [unwired: 1 in]
    n379 = Bundle("img_rows"="img_rows", "img_cols"="img_cols", "AT"="AT", "GB"="GB", "N_pts"="N_pts") -> (w991:T9)  [unwired: 1 in]
    n380 = call "Acquisition.vi"("uc480.Camera"=w1020, "Camera Param. Control Cluster"=w985, "Bits/Pixel in"=w1025, "Pupil Param. Calc. Data Cluster"=w991, "Error In"=w1028) -> ("uc480.Camera"=w1027:refnum<k24>, "Image To Save"=w1005:u8[][], "Framerate"=w997:dbl, "Camera Image"=→"Camera Image":picture, "Error Out"=w1026:errorcluster)  [unwired: 6 in]
    "Intensity graph output image" <- w1005
    n381 = Reciprocal(x=w997) -> (1/x=w1001:dbl)
    n382 = Multiply(x=w1001, y=1000.0) -> (x*y=w998:dbl)
    n383 = To Unsigned Long Integer(number=w998) -> (unsigned 32bit integer=w1000:u32)
    n384 = Wait Until Next ms Multiple(millisecond multiple=w1000) -> ()  [unwired: 1 out]
    n385 = property on="Intensity graph output image" class="IntGraph (strict)"() -> ("ZScale.Maximum"=w1004:dbl, "ZScale.Minimum"=w1003:dbl, "Color Table"=w1002:u32[])  [unwired: 2 in, 2 out]
    n386 = case shown="False" "Save image?" {
      tunnel: [w1030 w1041] -> w1015
      tunnel: [w1029 w1040] -> w1010
      tunnel: w1024 -> [w1030 w1039]
      tunnel: w1023 -> [w1029 w1038]
      tunnel: w1005 -> [_ w1034]
      tunnel: w1004 -> [_ w1033]
      tunnel: w1003 -> [_ w1032]
      tunnel: w1002 -> [_ w1031]
      frame False {
      }
      frame True {
        n387 = Get Date/Time In Seconds() -> (seconds since 1Jan1904=w1035:timestamp)
        n388 = Bundle(cluster=T4 {"Time stamp"=timestamp(0 s since 1904-01-01), "Image"=[], "Z Scale.Range:Maximum"=0.0, "Z Scale.Range:Minimum"=0.0, "Color Table"=[]}, "Time stamp"=w1035, "Image"=w1034, "Z Scale.Range:Maximum"=w1033, "Z Scale.Range:Minimum"=w1032, "Color Table"=w1031) -> (w1037:T4)
        n389 = Enqueue Element(queue=w1039, element=w1037, error in (no error)=w1038) -> (queue out=w1041:refnum<queue>, error out=w1040:errorcluster)  [unwired: 1 in, 1 out]
      }
    }
    n390 = property on="loop down cond." class="Bool (strict)"() -> (error out=w1007:errorcluster, "Value"=w1006:bool)  [unwired: 2 in, 1 out]
    n391 = Compound Arithmetic op=OR(w1010, w1026, w1016, "Stop program", w1007, w1006, w979) -> (w1008:bool)
    "loop up cond." <- w1008
    n392 = Get Queue Status(queue=w1015, error in (no error)=w1010) -> (queue out=w1022:refnum<queue>, error out=w1021:errorcluster, # elements in queue=w1014:i32)  [unwired: 1 in, 5 out]
    n393 = local write "#elements in queue"(w1014) -> ()
    n394 = Wait (ms)(milliseconds to wait=u32 3) -> ()  [unwired: 1 out]
  }
  n395 = flat-sequence {
    tunnel: w32 -> [w1044]
    tunnel: w31 -> [w1045]
    tunnel: w30 -> [w1081]
    tunnel: w29 -> [w1082]
    tunnel: w25 -> [w1108]
    tunnel: w24 -> [w1107]
    tunnel: w20 -> [w1106]
    tunnel: w19 -> [w1105]
    tunnel: w9 -> [w1104]
    tunnel: w12 -> [w1084]
    tunnel: w11 -> [w1083]
    tunnel: w1 -> [w1052]
    frame #0 {
      w1050 = T10 3 items=["no dialog", "OK message", "continue or stop message", "OK message + warnings", "continue/stop + warnings"] ("type of dialog (OK msg:1)")
      w1064 = T10 3 items=["no dialog", "OK message", "continue or stop message", "OK message + warnings", "continue/stop + warnings"] ("type of dialog (OK msg:1)")
      w1076 = T10 3 items=["no dialog", "OK message", "continue or stop message", "OK message + warnings", "continue/stop + warnings"] ("type of dialog (OK msg:1)")
      w1085 = T10 3 items=["no dialog", "OK message", "continue or stop message", "OK message + warnings", "continue/stop + warnings"] ("type of dialog (OK msg:1)")
      w1091 = T10 3 items=["no dialog", "OK message", "continue or stop message", "OK message + warnings", "continue/stop + warnings"] ("type of dialog (OK msg:1)")
      w1093 = T10 3 items=["no dialog", "OK message", "continue or stop message", "OK message + warnings", "continue/stop + warnings"] ("type of dialog (OK msg:1)")
      w1094 = T10 3 items=["no dialog", "OK message", "continue or stop message", "OK message + warnings", "continue/stop + warnings"] ("type of dialog (OK msg:1)")
      w1103 = T10 3 items=["no dialog", "OK message", "continue or stop message", "OK message + warnings", "continue/stop + warnings"] ("type of dialog (OK msg:1)")
      # "Scanners"
      # "Power Meter"
      # "Beep sound"
      # "Close PM"
      n396 = invoke on="Save image?" class="Bool (strict)" method="Reinit To Default"() -> ()  [unwired: 3 in, 3 out]
      n397 = invoke on="Stop program" class="Bool (strict)" method="Reinit To Default"() -> ()  [unwired: 3 in, 3 out]
      n398 = call "Close.vi"("error in (no error)"=w1107, "uc480.Camera"=w1108) -> ("error out"=w1077:errorcluster)  [unwired: 9 in]
      n399 = call <vilib>:"DAQmx Stop Task.vi"("task/channels in"=w1082, "error in"=w1081) -> ("task out"=w1099:refnum<k21>, "error out"=w1098:errorcluster)  [unwired: 12 in]
      "error out 2" <- w1098
      n400 = call "LEDs_OFF.vi"("channel"=w1052) -> ("error out"=w1059:errorcluster)  [unwired: 10 in]
      n401 = call <vilib>:"DAQmx Stop Task.vi"("task/channels in"=w1084, "error in"=w1083) -> ("task out"=w1096:refnum<k21>, "error out"=w1095:errorcluster)  [unwired: 12 in]
      n402 = call <vilib>:"Check if File or Folder Exists.vi"("path"="File Path") -> ("file or folder exists?"=w1074:bool, "dup path"=w1072:path)  [unwired: 8 in, 1 out]
      n403 = local read "Filter positions [deg]"() -> (w1043:sgl[])
      n404 = call "shutters_close.vi"("error in (no error)"=w1059, "channel"=w1052) -> ("error out"=w1058:errorcluster)  [unwired: 9 in]
      n405 = call <vilib>:"Simple Error Handler.vi"("type of dialog (OK msg:1)"=w1076, "error in (no error)"=w1077) -> ()  [unwired: 3 in, 5 out]
      n406 = call <vilib>:"DAQmx Clear Task.vi"("task in"=w1096, "error in"=w1095) -> ("error out"=w1097:errorcluster)  [unwired: 13 in]
      n407 = call "TLPMX Close.vi"("error in (no error)"=w1045, "instrument handle"=w1044) -> ("error out"=w1046:errorcluster)  [unwired: 9 in]
      n408 = call <vilib>:"DAQmx Clear Task.vi"("task in"=w1099, "error in"=w1098) -> ("error out"=w1080:errorcluster)  [unwired: 13 in]
      n409 = local read "Min/Max Voltage"() -> (w1067:dbl)
      n410 = local read "Number of trials k"() -> (w1062:i32)
      n411 = local read "Set Wavelength [nm]"() -> (w1068:dbl)
      n412 = local read "shiftX"() -> (w1066:dbl)
      n413 = local read "shiftY"() -> (w1065:dbl)
      n414 = local read "Answers"() -> (w1063:i32[][])
      n415 = call "GF_stop.vi"("modIdTag"="F1", "error in (no error)"=w1058, "channel"=w1052) -> ("error out"=w1057:errorcluster)  [unwired: 8 in]
      n416 = case shown="True" w1074 {
        tunnel: [path "F:/measdata" w1110] -> w1071
        tunnel: w1072 -> [_ w1110]
        frame False {
        }
        frame True {
        }
      }
      n417 = call <vilib>:"Simple Error Handler.vi"("type of dialog (OK msg:1)"=w1094, "error in (no error)"=w1097) -> ()  [unwired: 3 in, 5 out]
      n418 = call "GF_stop.vi"("modIdTag"="F2", "error in (no error)"=w1057, "channel"=w1052) -> ("error out"=w1054:errorcluster)  [unwired: 8 in]
      n419 = call <vilib>:"Clear Errors.vi"("error in (no error)"=w1080, "specific error code to clear (0: all)"=200010) -> ("error out"=w1079:errorcluster)  [unwired: 4 in, 1 out]
      n420 = Flush Queue(queue=w1106, error in (no error)=w1105) -> (queue out=w1090:refnum<queue>, remaining elements=w1075:T4[], error out=w1089:errorcluster)
      n421 = call <vilib>:"Simple Error Handler.vi"("type of dialog (OK msg:1)"=w1103, "error in (no error)"=w1046) -> ()  [unwired: 3 in, 5 out]
      n422 = call "LensMotor_stop.vi"("modIdTag"="S1", "error in (no error)"=w1054, "channel"=w1052) -> ("error out"=w1053:errorcluster)  [unwired: 8 in]
      n423 = To Double Precision Float(number=w1062) -> (double precision float=w1061:dbl)
      n424 = call "LensMotor_stop.vi"("modIdTag"="S2", "error in (no error)"=w1053, "channel"=w1052) -> ("error out"=w1060:errorcluster)  [unwired: 8 in]
      n425 = call <vilib>:"Simple Error Handler.vi"("type of dialog (OK msg:1)"=w1093, "error in (no error)"=w1079) -> ()  [unwired: 3 in, 5 out]
      n426 = Bundle("Set Wavelength [nm]"=w1068, "Min/Max Voltage"=w1067, "shiftX"=w1066, "shiftY"=w1065, "Filter positions [deg]"=w1043, "Answers"=w1063) -> (w1042:T11)  [unwired: 1 in]
      n427 = call "LensMotor_stop.vi"("modIdTag"="S3", "error in (no error)"=w1060, "channel"=w1052) -> ("error out"=w1051:errorcluster)  [unwired: 8 in]
      n428 = call <vilib>:"Beep.vi"("use system alert? (T)"=FALSE, "duration (msec)"=u32 50, "frequency (Hz)"=u32 523) -> ()  [unwired: 9 in]
      n429 = Release Queue(queue=w1090, error in (no error)=w1089) -> (error out=w1092:errorcluster)  [unwired: 1 in, 2 out]
      n430 = call <vilib>:"Simple Error Handler.vi"("type of dialog (OK msg:1)"=w1050, "error in (no error)"=w1051) -> ()  [unwired: 3 in, 5 out]
      n431 = call <vilib>:"Simple Error Handler.vi"("type of dialog (OK msg:1)"=w1091, "error in (no error)"=w1092) -> ()  [unwired: 3 in, 5 out]
      n432 = Path To String(path=w1071) -> (string=w1087:string)
      n433 = call "Save_meas_data.vi"("Path"=w1071, "Meas. Param. Data Cluster"=w1042, "Data"=w1104, "k"=w1061, "error in"=errorcluster {"status"=FALSE, "code"=0, "source"=""}) -> ("error out"=w1070:errorcluster)  [unwired: 10 in]
      n434 = call "Save_image.vi"("Path"=w1087, "remaining elements"=w1075) -> ("Number of saved images"=→"Number of saved images":i32, "error out"=w1086:errorcluster)  [unwired: 7 in]
      n435 = call <vilib>:"Simple Error Handler.vi"("type of dialog (OK msg:1)"=w1064, "error in (no error)"=w1070) -> ()  [unwired: 3 in, 5 out]
      n436 = call <vilib>:"Simple Error Handler.vi"("type of dialog (OK msg:1)"=w1085, "error in (no error)"=w1086) -> ()  [unwired: 3 in, 5 out]
    }
  }
